vi "Front End.vi"() -> ()   [LabVIEW 2026]
uses:
  <instrlib>/MicroPulse/Public/Data/Datatypes/MP - pulse damping.ctl
  <instrlib>/MicroPulse/Public/Data/Datatypes/MP - frequency filter.ctl
  <instrlib>/MicroPulse/Public/Data/Datatypes/MP - receive parameters.ctl
  <instrlib>/MicroPulse/Public/Data/Datatypes/MP - display gate.ctl
  <instrlib>/MicroPulse/Public/Data/Datatypes/MP - waveform type.ctl
  <instrlib>/MicroPulse/Public/Data/Datatypes/MP - analogue filter.ctl
  <instrlib>/MicroPulse/Public/Data/Datatypes/MP - digital filtering.ctl
  <instrlib>/MicroPulse/Public/Data/Datatypes/MP - high pass filter.ctl
  <instrlib>/MicroPulse/Public/Data/Datatypes/MP - low pass filter.ctl
  <instrlib>/MicroPulse/Public/Data/Datatypes/MP - multi-gate inspection.ctl
  <instrlib>/MicroPulse/Public/Data/Datatypes/MP - multigate inspection gate parameters.ctl
  <instrlib>/MicroPulse/Public/Data/Datatypes/MP - hysteresis level.ctl
  <instrlib>/MicroPulse/Public/Data/Datatypes/MP - multigate mode.ctl
  <instrlib>/MicroPulse/Public/Data/Datatypes/MP - data formatting.ctl
  <instrlib>/MicroPulse/Public/Data/Datatypes/MP - amplitude reporting mode.ctl
  <instrlib>/MicroPulse/Public/Data/Datatypes/MP - averaging.ctl
  <instrlib>/MicroPulse/Public/Data/Datatypes/MP - transmit parameters.ctl
  <instrlib>/MicroPulse/Public/Data/Datatypes/MP - pulser voltage.ctl
  <instrlib>/MicroPulse/Public/Data/Datatypes/TCP config.ctl
  <instrlib>/MicroPulse/Public/Data/Datatypes/MP - sample frequency.ctl
  <instrlib>/MicroPulse/Public/Data/Datatypes/MP - data output format.ctl
  <instrlib>/MicroPulse/Public/Data/Datatypes/MP - test parameters.ctl
  <vilib>/ErrorRing/Error Ring.xnode
  <instrlib>/MicroPulse/MicroPulse_Driver.lvlib
panel:
  in  "Main Tab Control":T1(tab)
  in  "Gain Slider":dbl(slide) caption="Gain (dB)" min=0.0 max=60.0 step=0.25 scale=0.0..60.0
  out "Channel Setup Graph":cluster{"timebase":dbl[], "data":u16[]}[](graph)
  in  "E-Stop Reset":bool
  out "Axis Controls":T2
  in  "Channel Setup Tab Control":enum32{"1", "2", "3", "4", "5", "6", "7"}(tab)
  out "Channel 1 WP/AMP/TOF":T3
  in  "Channel 1 Filter/Rectification/VoS":T5={"Filter"=enum."No change", "Enum"=enum."Rectified Signal", "Velocity of Sound"=6.12}
  in  "Channel 1 A-Scan Window":cluster{"Start":dbl, "Range":dbl}={"Start"=0.0, "Range"=10.0} {"Range" min=0.0 step=5.0; "Start" min=0.0 step=5.0}
  in  "Channel 1 Backwall Gate":T6 {"Threshold" min=0.0 max=100.0 step=1.0; "Length" min=0.0 step=1.0; "Start" min=0.0 step=1.0}
  in  "Channel 1 Flaw Gate":T6 {"Threshold" min=0.0 max=100.0 step=1.0; "Length" min=0.0 step=1.0; "Start" min=0.0 step=1.0}
  in  "Channel 1 Interface":T6 {"Threshold" min=0.0 max=100.0 step=1.0; "Length" min=0.0 step=1.0; "Start" min=0.0 step=1.0}
  in  "Channel 1 PW & DAMP":cluster{"Damping":T7, "Pulse Width":dbl}={"Damping"=enum."149W", "Pulse Width"=80.0} caption="Pulse Width & Damping 1" {"Pulse Width" step=1.0 format="%#_g ns"}
  in  "Channel 2 Filter/Rectification/VoS":T5
  out "Channel 2 WP/AMP/TOF":T3
  in  "Channel 2 A-Scan Window":cluster{"Start":dbl, "Range":dbl}={"Start"=0.0, "Range"=15.0} {"Range" min=0.0 step=1.0; "Start" min=0.0 step=1.0}
  in  "Channel 2 Backwall Gate":T6 {"Threshold" min=0.0 max=100.0 step=1.0; "Length" min=0.0 step=1.0; "Start" min=0.0 step=1.0}
  in  "Channel 2 Flaw Gate":T6 {"Threshold" min=0.0 max=100.0 step=1.0; "Length" min=0.0 step=1.0; "Start" min=0.0 step=1.0}
  in  "Channel 2 Interface":T6 {"Threshold" min=0.0 max=100.0 step=1.0; "Length" min=0.0 step=1.0; "Start" min=0.0 step=1.0}
  in  "Channel 2 PW & DAMP":cluster{"Damping":T7, "Pulse Width":dbl}={"Damping"=enum."149W", "Pulse Width"=80.0} caption="Pulse Width & Damping 1" {"Pulse Width" step=1.0 format="%#_g ns"}
  in  "Channel 3 PW & DAMP":cluster{"Damping":T7, "Pulse Width":dbl}={"Damping"=enum."149W", "Pulse Width"=80.0} caption="Pulse Width & Damping 1" {"Pulse Width" step=1.0 format="%#_g ns"}
  in  "Channel 3 Interface":T6 {"Threshold" min=0.0 max=100.0 step=1.0; "Length" min=0.0 step=1.0; "Start" min=0.0 step=1.0}
  in  "Channel 3 Flaw Gate":T6 {"Threshold" min=0.0 max=100.0 step=1.0; "Length" min=0.0 step=1.0; "Start" min=0.0 step=1.0}
  in  "Channel 3 Backwall Gate":T6 {"Threshold" min=0.0 max=100.0 step=1.0; "Length" min=0.0 step=1.0; "Start" min=0.0 step=1.0}
  in  "Channel 3 A-Scan Window":cluster{"Start":dbl, "Range":dbl}={"Start"=0.0, "Range"=20.0} {"Range" min=0.0 step=1.0; "Start" min=0.0 step=1.0}
  out "Channel 3 WP/AMP/TOF":T3
  in  "Channel 3 Filter/Rectification/VoS":T5
  in  "Channel 4 Filter/Rectification/VoS":T5
  in  "Channel 4 PW & DAMP":cluster{"Damping":T7, "Pulse Width":dbl}={"Damping"=enum."149W", "Pulse Width"=80.0} caption="Pulse Width & Damping 1" {"Pulse Width" step=1.0 format="%#_g ns"}
  in  "Channel 4 Interface":T6 {"Threshold" min=0.0 max=100.0 step=1.0; "Length" min=0.0 step=1.0; "Start" min=0.0 step=1.0}
  in  "Channel 4 Flaw Gate":T6 {"Threshold" min=0.0 max=100.0 step=1.0; "Length" min=0.0 step=1.0; "Start" min=0.0 step=1.0}
  in  "Channel 4 Backwall Gate":T6 {"Threshold" min=0.0 max=100.0 step=1.0; "Length" min=0.0 step=1.0; "Start" min=0.0 step=1.0}
  in  "Channel 4 A-Scan Window":cluster{"Start":dbl, "Range":dbl}={"Start"=0.0, "Range"=25.0} {"Range" min=0.0 step=1.0; "Start" min=0.0 step=1.0}
  out "Channel 4 WP/AMP/TOF":T3
  in  "Channel 5 Filter/Rectification/VoS":T5
  in  "Channel 5 PW & DAMP":cluster{"Damping":T7, "Pulse Width":dbl}={"Damping"=enum."149W", "Pulse Width"=80.0} caption="Pulse Width & Damping 1" {"Pulse Width" step=1.0 format="%#_g ns"}
  in  "Channel 5 Interface":T6 {"Threshold" min=0.0 max=100.0 step=1.0; "Length" min=0.0 step=1.0; "Start" min=0.0 step=1.0}
  in  "Channel 5 Flaw Gate":T6 {"Threshold" min=0.0 max=100.0 step=1.0; "Length" min=0.0 step=1.0; "Start" min=0.0 step=1.0}
  in  "Channel 5 Backwall Gate":T6 {"Threshold" min=0.0 max=100.0 step=1.0; "Length" min=0.0 step=1.0; "Start" min=0.0 step=1.0}
  in  "Channel 5 A-Scan Window":cluster{"Start":dbl, "Range":dbl}={"Start"=0.0, "Range"=30.0} {"Range" min=0.0 step=1.0; "Start" min=0.0 step=1.0}
  out "Channel 5 WP/AMP/TOF":T3
  in  "Channel 6 Filter/Rectification/VoS":T5
  in  "Channel 6 PW & DAMP":cluster{"Damping":T7, "Pulse Width":dbl}={"Damping"=enum."149W", "Pulse Width"=80.0} caption="Pulse Width & Damping 1" {"Pulse Width" step=1.0 format="%#_g ns"}
  in  "Channel 6 Interface":T6 {"Threshold" min=0.0 max=100.0 step=1.0; "Length" min=0.0 step=1.0; "Start" min=0.0 step=1.0}
  in  "Channel 6 Flaw Gate":T6 {"Threshold" min=0.0 max=100.0 step=1.0; "Length" min=0.0 step=1.0; "Start" min=0.0 step=1.0}
  in  "Channel 6 Backwall Gate":T6 {"Threshold" min=0.0 max=100.0 step=1.0; "Length" min=0.0 step=1.0; "Start" min=0.0 step=1.0}
  in  "Channel 6 A-Scan Window":cluster{"Start":dbl, "Range":dbl}={"Start"=0.0, "Range"=35.0} {"Range" min=0.0 step=1.0; "Start" min=0.0 step=1.0}
  out "Channel 6 WP/AMP/TOF":T3
  in  "Channel 7 Filter/Rectification/VoS":T5
  in  "Channel 7 PW & DAMP":cluster{"Damping":T7, "Pulse Width":dbl}={"Damping"=enum."149W", "Pulse Width"=80.0} caption="Pulse Width & Damping 1" {"Pulse Width" step=1.0 format="%#_g ns"}
  in  "Channel 7 Interface":T6 {"Threshold" min=0.0 max=100.0 step=1.0; "Length" min=0.0 step=1.0; "Start" min=0.0 step=1.0}
  in  "Channel 7 Flaw Gate":T6 {"Threshold" min=0.0 max=100.0 step=1.0; "Length" min=0.0 step=1.0; "Start" min=0.0 step=1.0}
  in  "Channel 7 Backwall Gate":T6 {"Threshold" min=0.0 max=100.0 step=1.0; "Length" min=0.0 step=1.0; "Start" min=0.0 step=1.0}
  in  "Channel 7 A-Scan Window":cluster{"Start":dbl, "Range":dbl}={"Start"=0.0, "Range"=40.0} {"Range" min=0.0 step=1.0; "Start" min=0.0 step=1.0}
  out "Channel 7 WP/AMP/TOF":T3
  in  "Channel Select":u16(ring) items=["Channel 1", "Channel 2", "Channel 3", "Channel 4", "Channel 5", "Channel 6", "Channel 7", "Channel 8", "Channel 9"]
  in  "MicroPulse Config Switch":u16(ring) items=["MicroPulse", "Channel 1", "Channel 2", "Channel 3", "Channel 4", "Channel 5", "Channel 6", "Channel 7", "Channel 8", "Channel 9"]
  in  "MicroPulse SysDiag Tab":T8(tab)
  in  "TCP config":T9={"Connection ID"=refnum, "IP address"="10.1.1.2", "host port"=1067, "OC timeout"=-1, "Read timeout"=0, "Write timeout"=0} {"Write timeout" format="%dms"; "Read timeout" format="%dms"; "OC timeout" format="%dms"}
  in  "Sample Frequency":T10
  in  "PRF (Hz)":dbl=50.0
  in  "Mode":T11=enum."8-bit Mode"
  in  "Receive Parameters 1":T12 {"Delay" format="%#_g us"; "Display Gate"."Length" min=0.0 max=64000.0 step=1.0 format="%#_g us"; "Display Gate"."Start" min=0.0 max=64000.0 step=1.0 format="%#_g us"; "Analogue Filtering"."Smoothing" min=1 max=11 step=1; "Gain" min=-6.0 max=70.0 step=0.25 format="%.2fdB"}
  in  "Multi Gate Inspection 1":T19={"Gate 1"={"Start (us)"=0.0, "Length (us)"=0.0, "Threshold"=10, "Enabled?"=TRUE, "Max # Peaks"=0, "Hysteresis"=enum."None", "Mode"=enum."1st Peak in Gate", "Inverted?"=FALSE, "Colour "=6618880}, "Gate 2"={"Start (us)"=0.0, "Length (us)"=0.0, "Threshold"=10, "Enabled?"=TRUE, "Max # Peaks"=0, "Hysteresis"=enum."None", "Mode"=enum."1st Peak in Gate", "Inverted?"=FALSE, "Colour "=16860}, "Gate 3"={"Start (us)"=0.0, "Length (us)"=0.0, "Threshold"=10, "Enabled?"=TRUE, "Max # Peaks"=0, "Hysteresis"=enum."None", "Mode"=enum."1st Peak in Gate", "Inverted?"=FALSE, "Colour "=16711680}, "Gate 4"={"Start (us)"=0.0, "Length (us)"=0.0, "Threshold"=10, "Enabled?"=FALSE, "Max # Peaks"=0, "Hysteresis"=enum."None", "Mode"=enum."1st Peak in Gate", "Inverted?"=FALSE, "Colour "=0}} {"Gate 4"."Max # Peaks" max=64000 step=100; "Gate 4"."Threshold" min=10 max=4095 step=10; "Gate 4"."Length (us)" min=0.0 max=96000.0 step=100.0; "Gate 4"."Start (us)" min=0.0 max=64000.0 step=100.0; "Gate 3"."Max # Peaks" max=64000 step=100; "Gate 3"."Threshold" min=10 max=4095 step=10; "Gate 3"."Length (us)" min=0.0 max=96000.0 step=100.0; "Gate 3"."Start (us)" min=0.0 max=64000.0 step=100.0; "Gate 2"."Max # Peaks" max=64000 step=100; "Gate 2"."Threshold" min=10 max=4095 step=10; "Gate 2"."Length (us)" min=0.0 max=96000.0 step=100.0; "Gate 2"."Start (us)" min=0.0 max=64000.0 step=100.0; "Gate 1"."Max # Peaks" max=64000 step=100; "Gate 1"."Threshold" min=10 max=4095 step=10; "Gate 1"."Length (us)" min=0.0 max=96000.0 step=100.0; "Gate 1"."Start (us)" min=0.0 max=64000.0 step=100.0}
  in  "Data Formatting 1":T23={"Amplitude Mode"=enum."Peaks + Ascan for Multigate", "Averaging"=enum."None", "Coupling Level"=0} {"Coupling Level" max=4095 step=1}
  in  "Transmit Parameters 1":T26 {"Pulse Shape"."Width" min=16 max=1010 step=50 format="%.0fns"}
  in  "Receive Parameters 2":T12 {"Delay" format="%#_g us"; "Display Gate"."Length" min=0.0 max=64000.0 step=1.0 format="%#_g us"; "Display Gate"."Start" min=0.0 max=64000.0 step=1.0 format="%#_g us"; "Analogue Filtering"."Smoothing" min=1 max=11 step=1; "Gain" min=-6.0 max=70.0 step=0.25 format="%.2fdB"}
  in  "Multi Gate Inspection 2":T19={"Gate 1"={"Start (us)"=0.0, "Length (us)"=0.0, "Threshold"=10, "Enabled?"=FALSE, "Max # Peaks"=0, "Hysteresis"=enum."None", "Mode"=enum."1st Peak in Gate", "Inverted?"=FALSE, "Colour "=0}, "Gate 2"={"Start (us)"=0.0, "Length (us)"=0.0, "Threshold"=10, "Enabled?"=FALSE, "Max # Peaks"=0, "Hysteresis"=enum."None", "Mode"=enum."1st Peak in Gate", "Inverted?"=FALSE, "Colour "=0}, "Gate 3"={"Start (us)"=0.0, "Length (us)"=0.0, "Threshold"=10, "Enabled?"=FALSE, "Max # Peaks"=0, "Hysteresis"=enum."None", "Mode"=enum."1st Peak in Gate", "Inverted?"=FALSE, "Colour "=0}, "Gate 4"={"Start (us)"=0.0, "Length (us)"=0.0, "Threshold"=10, "Enabled?"=FALSE, "Max # Peaks"=0, "Hysteresis"=enum."None", "Mode"=enum."1st Peak in Gate", "Inverted?"=FALSE, "Colour "=0}} {"Gate 4"."Max # Peaks" max=64000 step=100; "Gate 4"."Threshold" min=10 max=4095 step=10; "Gate 4"."Length (us)" min=0.0 max=96000.0 step=100.0; "Gate 4"."Start (us)" min=0.0 max=64000.0 step=100.0; "Gate 3"."Max # Peaks" max=64000 step=100; "Gate 3"."Threshold" min=10 max=4095 step=10; "Gate 3"."Length (us)" min=0.0 max=96000.0 step=100.0; "Gate 3"."Start (us)" min=0.0 max=64000.0 step=100.0; "Gate 2"."Max # Peaks" max=64000 step=100; "Gate 2"."Threshold" min=10 max=4095 step=10; "Gate 2"."Length (us)" min=0.0 max=96000.0 step=100.0; "Gate 2"."Start (us)" min=0.0 max=64000.0 step=100.0; "Gate 1"."Max # Peaks" max=64000 step=100; "Gate 1"."Threshold" min=10 max=4095 step=10; "Gate 1"."Length (us)" min=0.0 max=96000.0 step=100.0; "Gate 1"."Start (us)" min=0.0 max=64000.0 step=100.0}
  in  "Data Formatting 2":T23={"Amplitude Mode"=enum."Peaks + Ascan for Multigate", "Averaging"=enum."None", "Coupling Level"=0} {"Coupling Level" max=4095 step=1}
  in  "Transmit Parameters 2":T26 {"Pulse Shape"."Width" min=16 max=1010 step=50 format="%.0fns"}
  in  "Receive Parameters 3":T12 {"Delay" format="%#_g us"; "Display Gate"."Length" min=0.0 max=64000.0 step=1.0 format="%#_g us"; "Display Gate"."Start" min=0.0 max=64000.0 step=1.0 format="%#_g us"; "Analogue Filtering"."Smoothing" min=1 max=11 step=1; "Gain" min=-6.0 max=70.0 step=0.25 format="%.2fdB"}
  in  "Multi Gate Inspection 3":T19={"Gate 1"={"Start (us)"=0.0, "Length (us)"=0.0, "Threshold"=10, "Enabled?"=FALSE, "Max # Peaks"=0, "Hysteresis"=enum."None", "Mode"=enum."1st Peak in Gate", "Inverted?"=FALSE, "Colour "=0}, "Gate 2"={"Start (us)"=0.0, "Length (us)"=0.0, "Threshold"=10, "Enabled?"=FALSE, "Max # Peaks"=0, "Hysteresis"=enum."None", "Mode"=enum."1st Peak in Gate", "Inverted?"=FALSE, "Colour "=0}, "Gate 3"={"Start (us)"=0.0, "Length (us)"=0.0, "Threshold"=10, "Enabled?"=FALSE, "Max # Peaks"=0, "Hysteresis"=enum."None", "Mode"=enum."1st Peak in Gate", "Inverted?"=FALSE, "Colour "=0}, "Gate 4"={"Start (us)"=0.0, "Length (us)"=0.0, "Threshold"=10, "Enabled?"=FALSE, "Max # Peaks"=0, "Hysteresis"=enum."None", "Mode"=enum."1st Peak in Gate", "Inverted?"=FALSE, "Colour "=0}} {"Gate 4"."Max # Peaks" max=64000 step=100; "Gate 4"."Threshold" min=10 max=4095 step=10; "Gate 4"."Length (us)" min=0.0 max=96000.0 step=100.0; "Gate 4"."Start (us)" min=0.0 max=64000.0 step=100.0; "Gate 3"."Max # Peaks" max=64000 step=100; "Gate 3"."Threshold" min=10 max=4095 step=10; "Gate 3"."Length (us)" min=0.0 max=96000.0 step=100.0; "Gate 3"."Start (us)" min=0.0 max=64000.0 step=100.0; "Gate 2"."Max # Peaks" max=64000 step=100; "Gate 2"."Threshold" min=10 max=4095 step=10; "Gate 2"."Length (us)" min=0.0 max=96000.0 step=100.0; "Gate 2"."Start (us)" min=0.0 max=64000.0 step=100.0; "Gate 1"."Max # Peaks" max=64000 step=100; "Gate 1"."Threshold" min=10 max=4095 step=10; "Gate 1"."Length (us)" min=0.0 max=96000.0 step=100.0; "Gate 1"."Start (us)" min=0.0 max=64000.0 step=100.0}
  in  "Data Formatting 3":T23={"Amplitude Mode"=enum."Peaks + Ascan for Multigate", "Averaging"=enum."None", "Coupling Level"=0} {"Coupling Level" max=4095 step=1}
  in  "Transmit Parameters 3":T26 {"Pulse Shape"."Width" min=16 max=1010 step=50 format="%.0fns"}
  in  "Receive Parameters 4":T12 {"Delay" format="%#_g us"; "Display Gate"."Length" min=0.0 max=64000.0 step=1.0 format="%#_g us"; "Display Gate"."Start" min=0.0 max=64000.0 step=1.0 format="%#_g us"; "Analogue Filtering"."Smoothing" min=1 max=11 step=1; "Gain" min=-6.0 max=70.0 step=0.25 format="%.2fdB"}
  in  "Multi Gate Inspection 4":T19={"Gate 1"={"Start (us)"=0.0, "Length (us)"=0.0, "Threshold"=10, "Enabled?"=FALSE, "Max # Peaks"=0, "Hysteresis"=enum."None", "Mode"=enum."1st Peak in Gate", "Inverted?"=FALSE, "Colour "=0}, "Gate 2"={"Start (us)"=0.0, "Length (us)"=0.0, "Threshold"=10, "Enabled?"=FALSE, "Max # Peaks"=0, "Hysteresis"=enum."None", "Mode"=enum."1st Peak in Gate", "Inverted?"=FALSE, "Colour "=0}, "Gate 3"={"Start (us)"=0.0, "Length (us)"=0.0, "Threshold"=10, "Enabled?"=FALSE, "Max # Peaks"=0, "Hysteresis"=enum."None", "Mode"=enum."1st Peak in Gate", "Inverted?"=FALSE, "Colour "=0}, "Gate 4"={"Start (us)"=0.0, "Length (us)"=0.0, "Threshold"=10, "Enabled?"=FALSE, "Max # Peaks"=0, "Hysteresis"=enum."None", "Mode"=enum."1st Peak in Gate", "Inverted?"=FALSE, "Colour "=0}} {"Gate 4"."Max # Peaks" max=64000 step=100; "Gate 4"."Threshold" min=10 max=4095 step=10; "Gate 4"."Length (us)" min=0.0 max=96000.0 step=100.0; "Gate 4"."Start (us)" min=0.0 max=64000.0 step=100.0; "Gate 3"."Max # Peaks" max=64000 step=100; "Gate 3"."Threshold" min=10 max=4095 step=10; "Gate 3"."Length (us)" min=0.0 max=96000.0 step=100.0; "Gate 3"."Start (us)" min=0.0 max=64000.0 step=100.0; "Gate 2"."Max # Peaks" max=64000 step=100; "Gate 2"."Threshold" min=10 max=4095 step=10; "Gate 2"."Length (us)" min=0.0 max=96000.0 step=100.0; "Gate 2"."Start (us)" min=0.0 max=64000.0 step=100.0; "Gate 1"."Max # Peaks" max=64000 step=100; "Gate 1"."Threshold" min=10 max=4095 step=10; "Gate 1"."Length (us)" min=0.0 max=96000.0 step=100.0; "Gate 1"."Start (us)" min=0.0 max=64000.0 step=100.0}
  in  "Data Formatting 4":T23={"Amplitude Mode"=enum."Peaks + Ascan for Multigate", "Averaging"=enum."None", "Coupling Level"=0} {"Coupling Level" max=4095 step=1}
  in  "Transmit Parameters 4":T26 {"Pulse Shape"."Width" min=16 max=1010 step=50 format="%.0fns"}
  in  "Receive Parameters 5":T12 {"Delay" format="%#_g us"; "Display Gate"."Length" min=0.0 max=64000.0 step=1.0 format="%#_g us"; "Display Gate"."Start" min=0.0 max=64000.0 step=1.0 format="%#_g us"; "Analogue Filtering"."Smoothing" min=1 max=11 step=1; "Gain" min=-6.0 max=70.0 step=0.25 format="%.2fdB"}
  in  "Multi Gate Inspection 5":T19={"Gate 1"={"Start (us)"=0.0, "Length (us)"=0.0, "Threshold"=10, "Enabled?"=FALSE, "Max # Peaks"=0, "Hysteresis"=enum."None", "Mode"=enum."1st Peak in Gate", "Inverted?"=FALSE, "Colour "=0}, "Gate 2"={"Start (us)"=0.0, "Length (us)"=0.0, "Threshold"=10, "Enabled?"=FALSE, "Max # Peaks"=0, "Hysteresis"=enum."None", "Mode"=enum."1st Peak in Gate", "Inverted?"=FALSE, "Colour "=0}, "Gate 3"={"Start (us)"=0.0, "Length (us)"=0.0, "Threshold"=10, "Enabled?"=FALSE, "Max # Peaks"=0, "Hysteresis"=enum."None", "Mode"=enum."1st Peak in Gate", "Inverted?"=FALSE, "Colour "=0}, "Gate 4"={"Start (us)"=0.0, "Length (us)"=0.0, "Threshold"=10, "Enabled?"=FALSE, "Max # Peaks"=0, "Hysteresis"=enum."None", "Mode"=enum."1st Peak in Gate", "Inverted?"=FALSE, "Colour "=0}} {"Gate 4"."Max # Peaks" max=64000 step=100; "Gate 4"."Threshold" min=10 max=4095 step=10; "Gate 4"."Length (us)" min=0.0 max=96000.0 step=100.0; "Gate 4"."Start (us)" min=0.0 max=64000.0 step=100.0; "Gate 3"."Max # Peaks" max=64000 step=100; "Gate 3"."Threshold" min=10 max=4095 step=10; "Gate 3"."Length (us)" min=0.0 max=96000.0 step=100.0; "Gate 3"."Start (us)" min=0.0 max=64000.0 step=100.0; "Gate 2"."Max # Peaks" max=64000 step=100; "Gate 2"."Threshold" min=10 max=4095 step=10; "Gate 2"."Length (us)" min=0.0 max=96000.0 step=100.0; "Gate 2"."Start (us)" min=0.0 max=64000.0 step=100.0; "Gate 1"."Max # Peaks" max=64000 step=100; "Gate 1"."Threshold" min=10 max=4095 step=10; "Gate 1"."Length (us)" min=0.0 max=96000.0 step=100.0; "Gate 1"."Start (us)" min=0.0 max=64000.0 step=100.0}
  in  "Data Formatting 5":T23={"Amplitude Mode"=enum."Peaks + Ascan for Multigate", "Averaging"=enum."None", "Coupling Level"=0} {"Coupling Level" max=4095 step=1}
  in  "Transmit Parameters 5":T26 {"Pulse Shape"."Width" min=16 max=1010 step=50 format="%.0fns"}
  in  "Receive Parameters 6":T12 {"Delay" format="%#_g us"; "Display Gate"."Length" min=0.0 max=64000.0 step=1.0 format="%#_g us"; "Display Gate"."Start" min=0.0 max=64000.0 step=1.0 format="%#_g us"; "Analogue Filtering"."Smoothing" min=1 max=11 step=1; "Gain" min=-6.0 max=70.0 step=0.25 format="%.2fdB"}
  in  "Multi Gate Inspection 6":T19={"Gate 1"={"Start (us)"=0.0, "Length (us)"=0.0, "Threshold"=10, "Enabled?"=FALSE, "Max # Peaks"=0, "Hysteresis"=enum."None", "Mode"=enum."1st Peak in Gate", "Inverted?"=FALSE, "Colour "=0}, "Gate 2"={"Start (us)"=0.0, "Length (us)"=0.0, "Threshold"=10, "Enabled?"=FALSE, "Max # Peaks"=0, "Hysteresis"=enum."None", "Mode"=enum."1st Peak in Gate", "Inverted?"=FALSE, "Colour "=0}, "Gate 3"={"Start (us)"=0.0, "Length (us)"=0.0, "Threshold"=10, "Enabled?"=FALSE, "Max # Peaks"=0, "Hysteresis"=enum."None", "Mode"=enum."1st Peak in Gate", "Inverted?"=FALSE, "Colour "=0}, "Gate 4"={"Start (us)"=0.0, "Length (us)"=0.0, "Threshold"=10, "Enabled?"=FALSE, "Max # Peaks"=0, "Hysteresis"=enum."None", "Mode"=enum."1st Peak in Gate", "Inverted?"=FALSE, "Colour "=0}} {"Gate 4"."Max # Peaks" max=64000 step=100; "Gate 4"."Threshold" min=10 max=4095 step=10; "Gate 4"."Length (us)" min=0.0 max=96000.0 step=100.0; "Gate 4"."Start (us)" min=0.0 max=64000.0 step=100.0; "Gate 3"."Max # Peaks" max=64000 step=100; "Gate 3"."Threshold" min=10 max=4095 step=10; "Gate 3"."Length (us)" min=0.0 max=96000.0 step=100.0; "Gate 3"."Start (us)" min=0.0 max=64000.0 step=100.0; "Gate 2"."Max # Peaks" max=64000 step=100; "Gate 2"."Threshold" min=10 max=4095 step=10; "Gate 2"."Length (us)" min=0.0 max=96000.0 step=100.0; "Gate 2"."Start (us)" min=0.0 max=64000.0 step=100.0; "Gate 1"."Max # Peaks" max=64000 step=100; "Gate 1"."Threshold" min=10 max=4095 step=10; "Gate 1"."Length (us)" min=0.0 max=96000.0 step=100.0; "Gate 1"."Start (us)" min=0.0 max=64000.0 step=100.0}
  in  "Data Formatting 6":T23={"Amplitude Mode"=enum."Peaks + Ascan for Multigate", "Averaging"=enum."None", "Coupling Level"=0} {"Coupling Level" max=4095 step=1}
  in  "Transmit Parameters 6":T26 {"Pulse Shape"."Width" min=16 max=1010 step=50 format="%.0fns"}
  in  "Receive Parameters 7":T12 {"Delay" format="%#_g us"; "Display Gate"."Length" min=0.0 max=64000.0 step=1.0 format="%#_g us"; "Display Gate"."Start" min=0.0 max=64000.0 step=1.0 format="%#_g us"; "Analogue Filtering"."Smoothing" min=1 max=11 step=1; "Gain" min=-6.0 max=70.0 step=0.25 format="%.2fdB"}
  in  "Multi Gate Inspection 7":T19={"Gate 1"={"Start (us)"=0.0, "Length (us)"=0.0, "Threshold"=10, "Enabled?"=FALSE, "Max # Peaks"=0, "Hysteresis"=enum."None", "Mode"=enum."1st Peak in Gate", "Inverted?"=FALSE, "Colour "=0}, "Gate 2"={"Start (us)"=0.0, "Length (us)"=0.0, "Threshold"=10, "Enabled?"=FALSE, "Max # Peaks"=0, "Hysteresis"=enum."None", "Mode"=enum."1st Peak in Gate", "Inverted?"=FALSE, "Colour "=0}, "Gate 3"={"Start (us)"=0.0, "Length (us)"=0.0, "Threshold"=10, "Enabled?"=FALSE, "Max # Peaks"=0, "Hysteresis"=enum."None", "Mode"=enum."1st Peak in Gate", "Inverted?"=FALSE, "Colour "=0}, "Gate 4"={"Start (us)"=0.0, "Length (us)"=0.0, "Threshold"=10, "Enabled?"=FALSE, "Max # Peaks"=0, "Hysteresis"=enum."None", "Mode"=enum."1st Peak in Gate", "Inverted?"=FALSE, "Colour "=0}} {"Gate 4"."Max # Peaks" max=64000 step=100; "Gate 4"."Threshold" min=10 max=4095 step=10; "Gate 4"."Length (us)" min=0.0 max=96000.0 step=100.0; "Gate 4"."Start (us)" min=0.0 max=64000.0 step=100.0; "Gate 3"."Max # Peaks" max=64000 step=100; "Gate 3"."Threshold" min=10 max=4095 step=10; "Gate 3"."Length (us)" min=0.0 max=96000.0 step=100.0; "Gate 3"."Start (us)" min=0.0 max=64000.0 step=100.0; "Gate 2"."Max # Peaks" max=64000 step=100; "Gate 2"."Threshold" min=10 max=4095 step=10; "Gate 2"."Length (us)" min=0.0 max=96000.0 step=100.0; "Gate 2"."Start (us)" min=0.0 max=64000.0 step=100.0; "Gate 1"."Max # Peaks" max=64000 step=100; "Gate 1"."Threshold" min=10 max=4095 step=10; "Gate 1"."Length (us)" min=0.0 max=96000.0 step=100.0; "Gate 1"."Start (us)" min=0.0 max=64000.0 step=100.0}
  in  "Data Formatting 7":T23={"Amplitude Mode"=enum."Peaks + Ascan for Multigate", "Averaging"=enum."None", "Coupling Level"=0} {"Coupling Level" max=4095 step=1}
  in  "Transmit Parameters 7":T26 {"Pulse Shape"."Width" min=16 max=1010 step=50 format="%.0fns"}
  in  "Receive Parameters 8":T12 {"Delay" format="%#_g us"; "Display Gate"."Length" min=0.0 max=64000.0 step=1.0 format="%#_g us"; "Display Gate"."Start" min=0.0 max=64000.0 step=1.0 format="%#_g us"; "Analogue Filtering"."Smoothing" min=1 max=11 step=1; "Gain" min=-6.0 max=70.0 step=0.25 format="%.2fdB"}
  in  "Multi Gate Inspection 8":T19={"Gate 1"={"Start (us)"=0.0, "Length (us)"=0.0, "Threshold"=10, "Enabled?"=FALSE, "Max # Peaks"=0, "Hysteresis"=enum."None", "Mode"=enum."1st Peak in Gate", "Inverted?"=FALSE, "Colour "=0}, "Gate 2"={"Start (us)"=0.0, "Length (us)"=0.0, "Threshold"=10, "Enabled?"=FALSE, "Max # Peaks"=0, "Hysteresis"=enum."None", "Mode"=enum."1st Peak in Gate", "Inverted?"=FALSE, "Colour "=0}, "Gate 3"={"Start (us)"=0.0, "Length (us)"=0.0, "Threshold"=10, "Enabled?"=FALSE, "Max # Peaks"=0, "Hysteresis"=enum."None", "Mode"=enum."1st Peak in Gate", "Inverted?"=FALSE, "Colour "=0}, "Gate 4"={"Start (us)"=0.0, "Length (us)"=0.0, "Threshold"=10, "Enabled?"=FALSE, "Max # Peaks"=0, "Hysteresis"=enum."None", "Mode"=enum."1st Peak in Gate", "Inverted?"=FALSE, "Colour "=0}} {"Gate 4"."Max # Peaks" max=64000 step=100; "Gate 4"."Threshold" min=10 max=4095 step=10; "Gate 4"."Length (us)" min=0.0 max=96000.0 step=100.0; "Gate 4"."Start (us)" min=0.0 max=64000.0 step=100.0; "Gate 3"."Max # Peaks" max=64000 step=100; "Gate 3"."Threshold" min=10 max=4095 step=10; "Gate 3"."Length (us)" min=0.0 max=96000.0 step=100.0; "Gate 3"."Start (us)" min=0.0 max=64000.0 step=100.0; "Gate 2"."Max # Peaks" max=64000 step=100; "Gate 2"."Threshold" min=10 max=4095 step=10; "Gate 2"."Length (us)" min=0.0 max=96000.0 step=100.0; "Gate 2"."Start (us)" min=0.0 max=64000.0 step=100.0; "Gate 1"."Max # Peaks" max=64000 step=100; "Gate 1"."Threshold" min=10 max=4095 step=10; "Gate 1"."Length (us)" min=0.0 max=96000.0 step=100.0; "Gate 1"."Start (us)" min=0.0 max=64000.0 step=100.0}
  in  "Data Formatting 8":T23={"Amplitude Mode"=enum."Peaks + Ascan for Multigate", "Averaging"=enum."None", "Coupling Level"=0} {"Coupling Level" max=4095 step=1}
  in  "Transmit Parameters 8":T26 {"Pulse Shape"."Width" min=16 max=1010 step=50 format="%.0fns"}
  in  "Receive Parameters 9":T12 {"Delay" format="%#_g us"; "Display Gate"."Length" min=0.0 max=64000.0 step=1.0 format="%#_g us"; "Display Gate"."Start" min=0.0 max=64000.0 step=1.0 format="%#_g us"; "Analogue Filtering"."Smoothing" min=1 max=11 step=1; "Gain" min=-6.0 max=70.0 step=0.25 format="%.2fdB"}
  in  "Multi Gate Inspection 9":T19={"Gate 1"={"Start (us)"=0.0, "Length (us)"=0.0, "Threshold"=10, "Enabled?"=FALSE, "Max # Peaks"=0, "Hysteresis"=enum."None", "Mode"=enum."1st Peak in Gate", "Inverted?"=FALSE, "Colour "=0}, "Gate 2"={"Start (us)"=0.0, "Length (us)"=0.0, "Threshold"=10, "Enabled?"=FALSE, "Max # Peaks"=0, "Hysteresis"=enum."None", "Mode"=enum."1st Peak in Gate", "Inverted?"=FALSE, "Colour "=0}, "Gate 3"={"Start (us)"=0.0, "Length (us)"=0.0, "Threshold"=10, "Enabled?"=FALSE, "Max # Peaks"=0, "Hysteresis"=enum."None", "Mode"=enum."1st Peak in Gate", "Inverted?"=FALSE, "Colour "=0}, "Gate 4"={"Start (us)"=0.0, "Length (us)"=0.0, "Threshold"=10, "Enabled?"=FALSE, "Max # Peaks"=0, "Hysteresis"=enum."None", "Mode"=enum."1st Peak in Gate", "Inverted?"=FALSE, "Colour "=0}} {"Gate 4"."Max # Peaks" max=64000 step=100; "Gate 4"."Threshold" min=10 max=4095 step=10; "Gate 4"."Length (us)" min=0.0 max=96000.0 step=100.0; "Gate 4"."Start (us)" min=0.0 max=64000.0 step=100.0; "Gate 3"."Max # Peaks" max=64000 step=100; "Gate 3"."Threshold" min=10 max=4095 step=10; "Gate 3"."Length (us)" min=0.0 max=96000.0 step=100.0; "Gate 3"."Start (us)" min=0.0 max=64000.0 step=100.0; "Gate 2"."Max # Peaks" max=64000 step=100; "Gate 2"."Threshold" min=10 max=4095 step=10; "Gate 2"."Length (us)" min=0.0 max=96000.0 step=100.0; "Gate 2"."Start (us)" min=0.0 max=64000.0 step=100.0; "Gate 1"."Max # Peaks" max=64000 step=100; "Gate 1"."Threshold" min=10 max=4095 step=10; "Gate 1"."Length (us)" min=0.0 max=96000.0 step=100.0; "Gate 1"."Start (us)" min=0.0 max=64000.0 step=100.0}
  in  "Data Formatting 9":T23={"Amplitude Mode"=enum."Peaks + Ascan for Multigate", "Averaging"=enum."None", "Coupling Level"=0} {"Coupling Level" max=4095 step=1}
  in  "Transmit Parameters 9":T26 {"Pulse Shape"."Width" min=16 max=1010 step=50 format="%.0fns"}
  in  "stop":bool
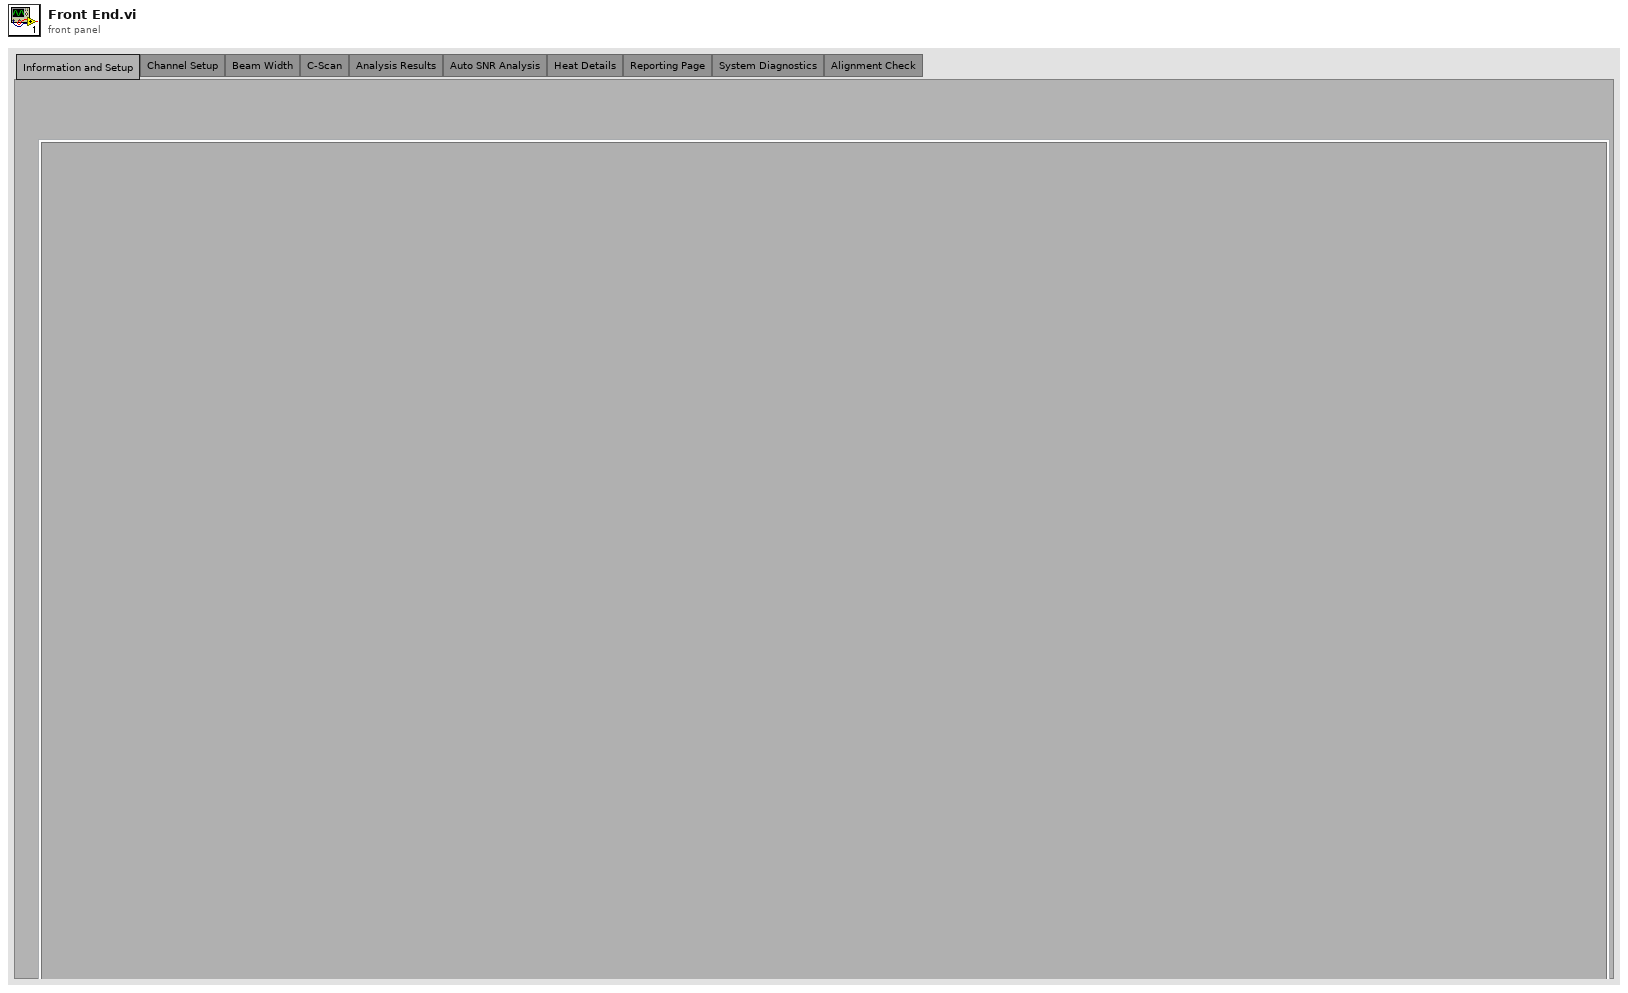
[diagram p1: front panel]
types:
  T1 = enum32{"Information and Setup", "Channel Setup", "Beam Width", "C-Scan", "Analysis Results", "Auto SNR Analysis", "Heat Details", "Reporting Page", "System Diagnostics", "Alignment Check"}
  T2 = cluster{"Buttons":cluster{"Datum":bool, "Move to Bar":bool, "Move to Home":bool}, "X Axis":cluster{"Calculated X Value":dbl, "Encoder X Value":dbl, "X Axis Movement Buttons":cluster{"Left":bool, "Right":bool, "Go To":bool, "Stop":bool}}, "Y Axis":cluster{"Encoder Y Value":dbl, "Y Axis Movement Buttons":cluster{"Left":bool, "Right":bool, "Go To":bool, "Stop":bool}, "Z Axis":cluster{"Encoder Z Value":dbl, "Z Axis Movement Buttons":cluster{"Left":bool, "Right":bool, "Go To":bool, "Stop":bool}}, "Rotate Axis":cluster{"Calculated Rotate Value":dbl, "Encoder Rotate Value":dbl, "Rotate Axis Movement Buttons":cluster{"Left":bool, "Right":bool, "Go To":bool, "Stop":bool}}, "Pitch Axis":cluster{"Encoder Pitch Value":dbl, "Pitch Axis Movement Buttons":cluster{"Left":bool, "Right":bool, "Go To":bool, "Stop":bool}}, "Roll Axis":cluster{"Encoder Roll Value":dbl, "Roll Axis Movement Buttons":cluster{"Left":bool, "Right":bool, "Go To":bool, "Stop":bool}}}}
  T3 = cluster{"Water Path":dbl, "Gate Amplitude":dbl, "Gate TOF":dbl}
  T4 = typedef "MicroPulse_Driver.lvlib/MP - frequency filter.ctl" = enum16{"No change", "1MHz Bandpass", "2MHz Bandpass", "4MHz Bandpass", "5MHz Bandpass", "10MHz Bandpass", "2.5-18MHz Broadband", "0.75-12MHz  Broadband", "0.5MHz Bandpass", "5MHz 2nd Order TOFD", "10MHz 2nd Order TOFD", "3.0-25MHz Broadband", "3.0-30MHz Broadband"}
  T5 = cluster{"Filter":T4, "Enum":enum16{"Rectified Signal", "RF Signal", "+Half Wave", "-Half Wave"}, "Velocity of Sound":dbl}
  T6 = cluster{"Start":dbl, "Length":dbl, "Threshold":dbl}
  T7 = typedef "MicroPulse_Driver.lvlib/MP - pulse damping.ctl" = enum16{"660W", "458W", "220W", "149W", "102W", "82W", "63W", "51W"}
  T8 = enum32{"MicroPulse", "Channel 1", "Channel 2", "Channel 3", "Channel 4", "Channel 5", "Channel 6", "Channel 7", "Channel 8", "Channel 9"}
  T9 = typedef "MicroPulse_Driver.lvlib/TCP config.ctl" = cluster{"Connection ID":refnum<k5>, "IP address":string, "host port":u16, "OC timeout":i32, "Read timeout":i32, "Write timeout":i32}
  T10 = typedef "MicroPulse_Driver.lvlib/MP - sample frequency.ctl" = enum16{"Use Default", "200MHz (LT2 only)", "100MHz", "50MHz", "25MHz", "10MHz"}
  T11 = typedef "MicroPulse_Driver.lvlib/MP - data output format.ctl" = enum16{"", "8-bit Mode", "10-bit Mode", "12-bit Mode", "16-bit Mode", "8-bit Log Mode", "12-bit Packed Mode"}
  T12 = typedef "MicroPulse_Driver.lvlib/MP - receive parameters.ctl" = cluster{"Display Gate":T13, "Delay":dbl, "Waveform Type":T14, "Gain":dbl, "Analogue Filtering":T15, "Digital Filtering":T16}
  T13 = typedef "MicroPulse_Driver.lvlib/MP - display gate.ctl" = cluster{"Start":dbl, "Length":dbl}
  T14 = typedef "MicroPulse_Driver.lvlib/MP - waveform type.ctl" = enum16{"Rectified Signal", "RF Signal", "+Half Wave", "-Half Wave"}
  T15 = typedef "MicroPulse_Driver.lvlib/MP - analogue filter.ctl" = cluster{"Bandpass":T4, "Smoothing":u16}
  T16 = typedef "MicroPulse_Driver.lvlib/MP - digital filtering.ctl" = cluster{"High Pass Filter":T17, "Low Pass Filter":T18}
  T17 = typedef "MicroPulse_Driver.lvlib/MP - high pass filter.ctl" = enum16{"None", "0.7MHz", "1.5MHz", "4.0MHz", "7.5MHz", "10.0MHz", "User Defined"}
  T18 = typedef "MicroPulse_Driver.lvlib/MP - low pass filter.ctl" = enum16{"None", "1.8MHz", "3.0MHz", "6.0MHz", "8.0MHz", "12.0MHz", "User Defined"}
  T19 = typedef "MicroPulse_Driver.lvlib/MP - multi-gate inspection.ctl" = cluster{"Gate 1":T20, "Gate 2":T20, "Gate 3":T20, "Gate 4":T20}
  T20 = typedef "MicroPulse_Driver.lvlib/MP - multigate inspection gate parameters.ctl" = cluster{"Start (us)":dbl, "Length (us)":dbl, "Threshold":u16, "Enabled?":bool, "Max # Peaks":u16, "Hysteresis":T21, "Mode":T22, "Inverted?":bool, "Colour ":u32}
  T21 = typedef "MicroPulse_Driver.lvlib/MP - hysteresis level.ctl" = enum16{"None", "3dB", "6dB", "9dB", "12dB"}
  T22 = typedef "MicroPulse_Driver.lvlib/MP - multigate mode.ctl" = enum16{"1st Peak in Gate", "Largest Peak In Gate", "All Peaks In Gate", "1st Threshold Crossing"}
  T23 = typedef "MicroPulse_Driver.lvlib/MP - data formatting.ctl" = cluster{"Amplitude Mode":T24, "Averaging":T25, "Coupling Level":u32}
  T24 = typedef "MicroPulse_Driver.lvlib/MP - amplitude reporting mode.ctl" = enum16{"1st Peak in gate", "Maximum Peak in gate", "All Peaks", "Ascan Data", "1st Threshold Crossing Peak", "Ascan + Peaks", "All Peaks for Multigate", "Peaks + Ascan for Multigate", "Peaks + P_Ascan for Multigate", "Full Matrix Capture"}
  T25 = typedef "MicroPulse_Driver.lvlib/MP - averaging.ctl" = enum16{"None", "2", "4", "8", "16", "32", "64", "128", "256"}
  T26 = typedef "MicroPulse_Driver.lvlib/MP - transmit parameters.ctl" = cluster{"Pulse Voltage":T27, "Pulse Shape":cluster{"Damping":T7, "Width":u32}}
  T27 = typedef "MicroPulse_Driver.lvlib/MP - pulser voltage.ctl" = enum16{"50V", "100V", "150V", "200V", "250V", "300V"}
  T28 = enum16{"Channel 1", "Channel 2", "Channel 3", "Channel 4", "Channel 5", "Channel 6", "Channel 7", "Channel 8", "Channel 9"}
  T29 = enum16{"Init", "Init HW", "Main", "Error", "Shutdown"}
  T30 = typedef "MicroPulse_Driver.lvlib/MP - test parameters.ctl" = cluster{"Test No.":u32, "Tx Channel":u32, "Rx Channel":u32}
  T31 = enum16{"Rectified Signal", "RF Signal", "+Half Wave", "-Half Wave"}
  T32 = typedef "MicroPulse_Driver.lvlib/MP - scan data info.ctl" = cluster{"Message Header":u16, "Error Message":u16, "Test No.":u32, "Channel No.":u8, "Sweep No.":u32, "Gate No.":u32, "DOF":T11, "retain data":T33, "scan data":u16[], "scan length":i32, "scan index":i32, "peak data":cluster{"timebase":u16[], "data":u16[]}, "#peaks":i32, "PRF":dbl, "IP":cluster{"Axis No.":u8, "Location":u32, "MIP location":u32, "MIP?":bool}, "echo range":u16, "ETG":bool, "CAL 0 complete":bool, "Axis Positions":T34}
  T33 = typedef "MicroPulse_Driver.lvlib/MP - retain scan.ctl" = enum16{"None", "Ascan", "Peaks"}
  T34 = typedef "MicroPulse_Driver.lvlib/MP - axis positions (LLC).ctl" = cluster{"Axis 1":u32, "Axis 2":u32, "Axis 3":u32, "Axis 4":u32, "Status":u8}
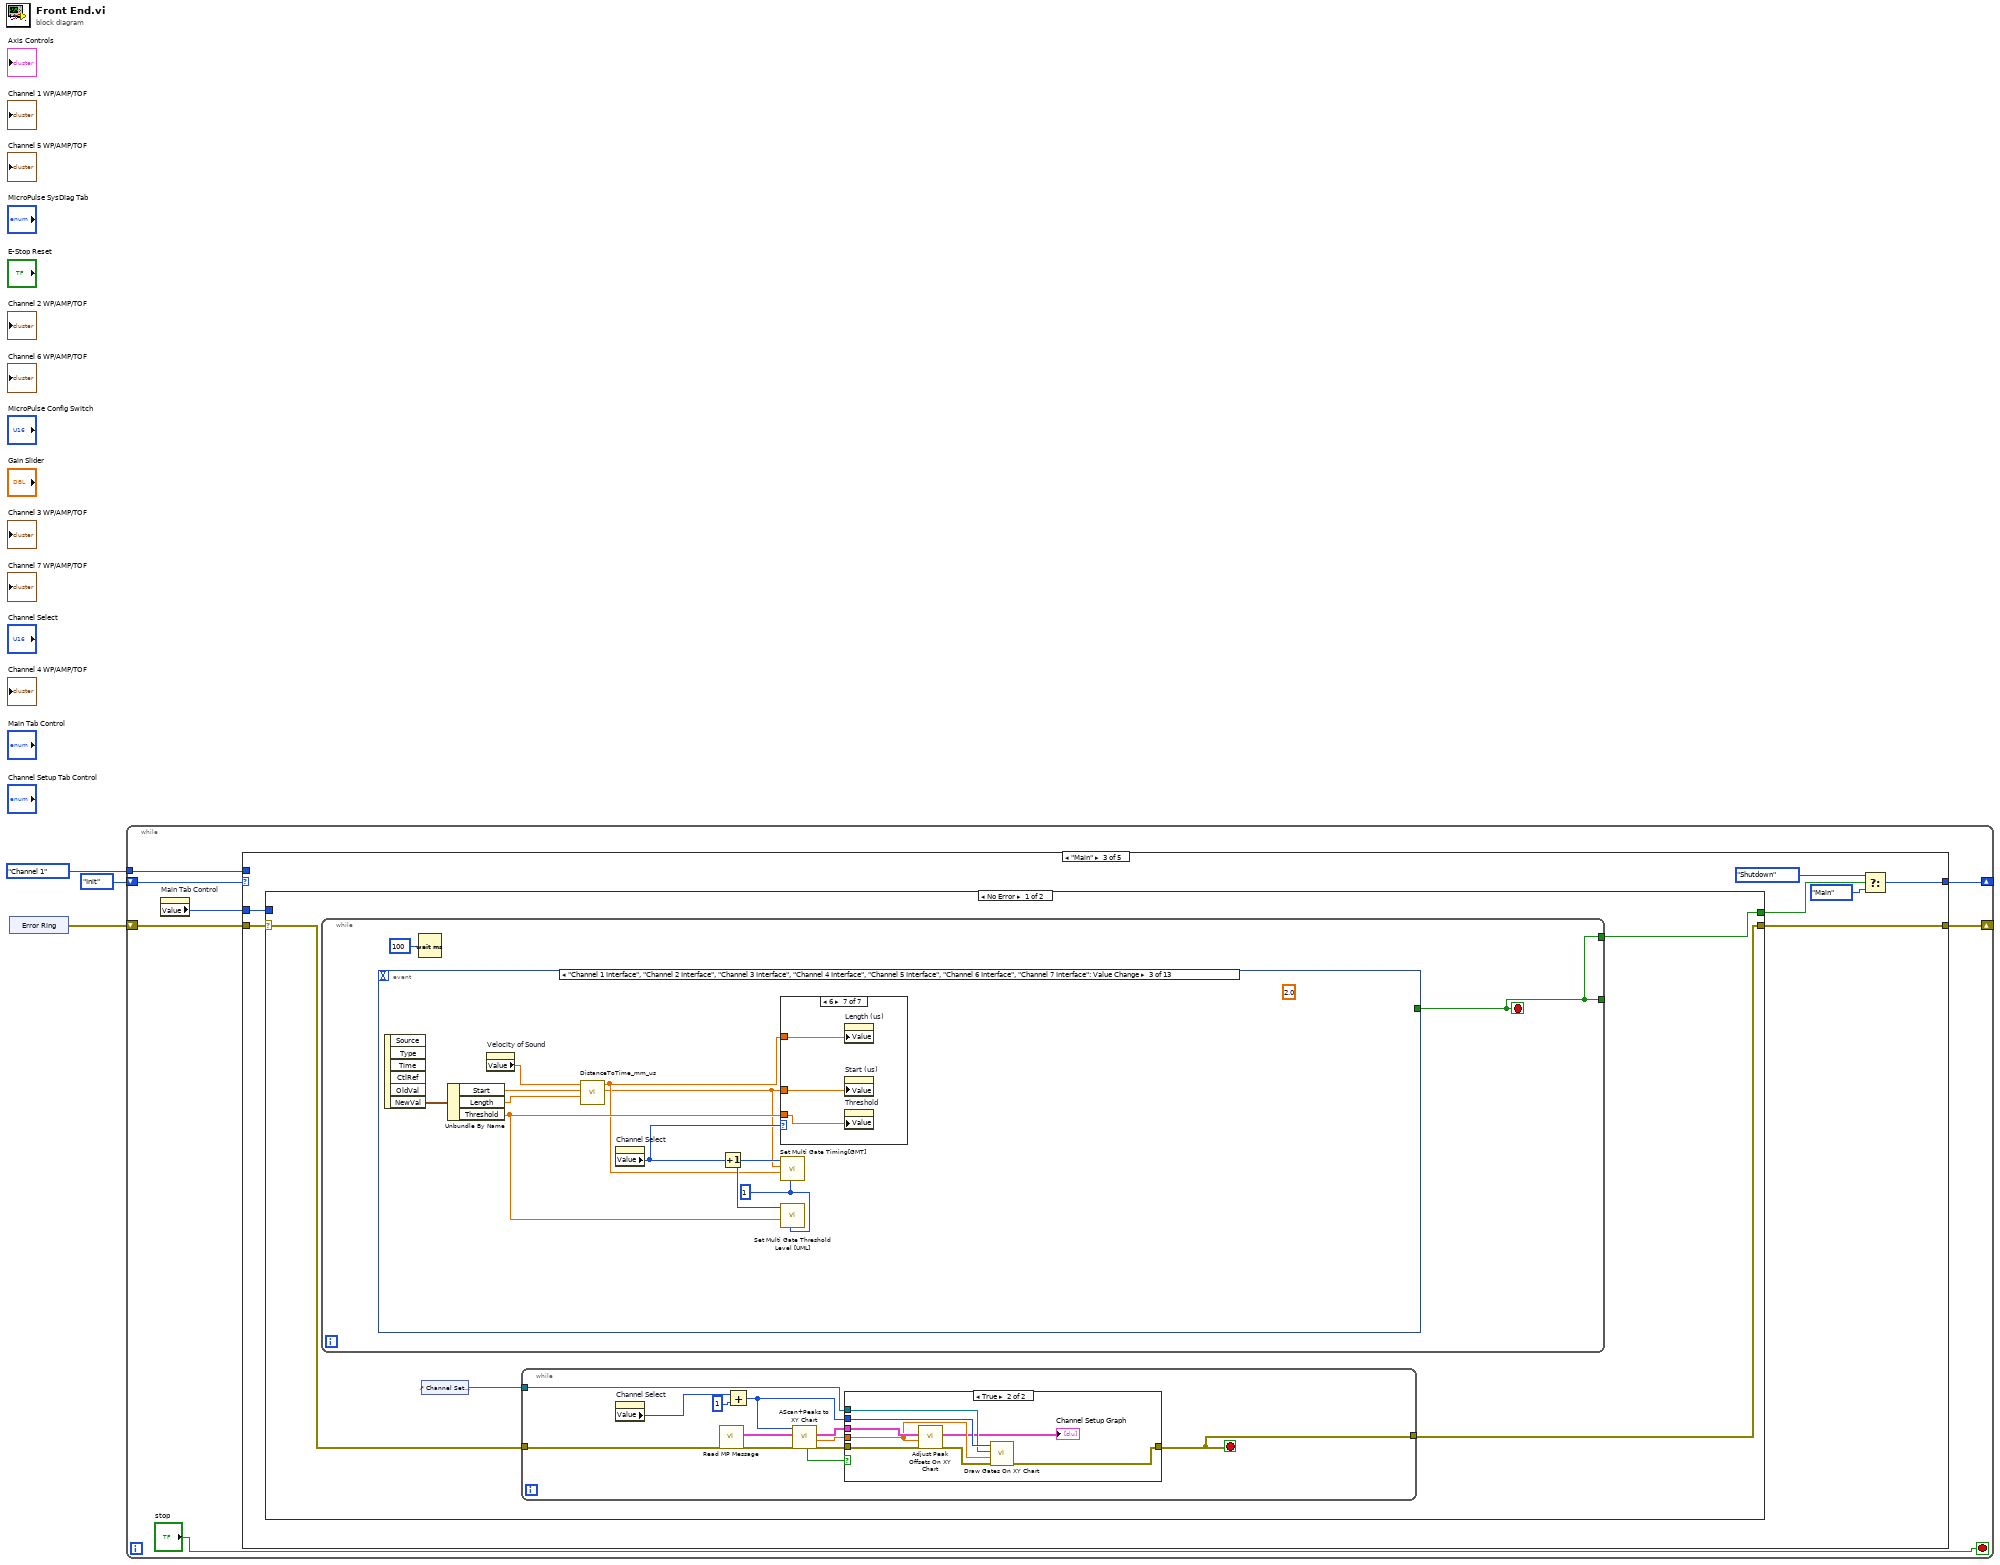
[diagram p0: block diagram]
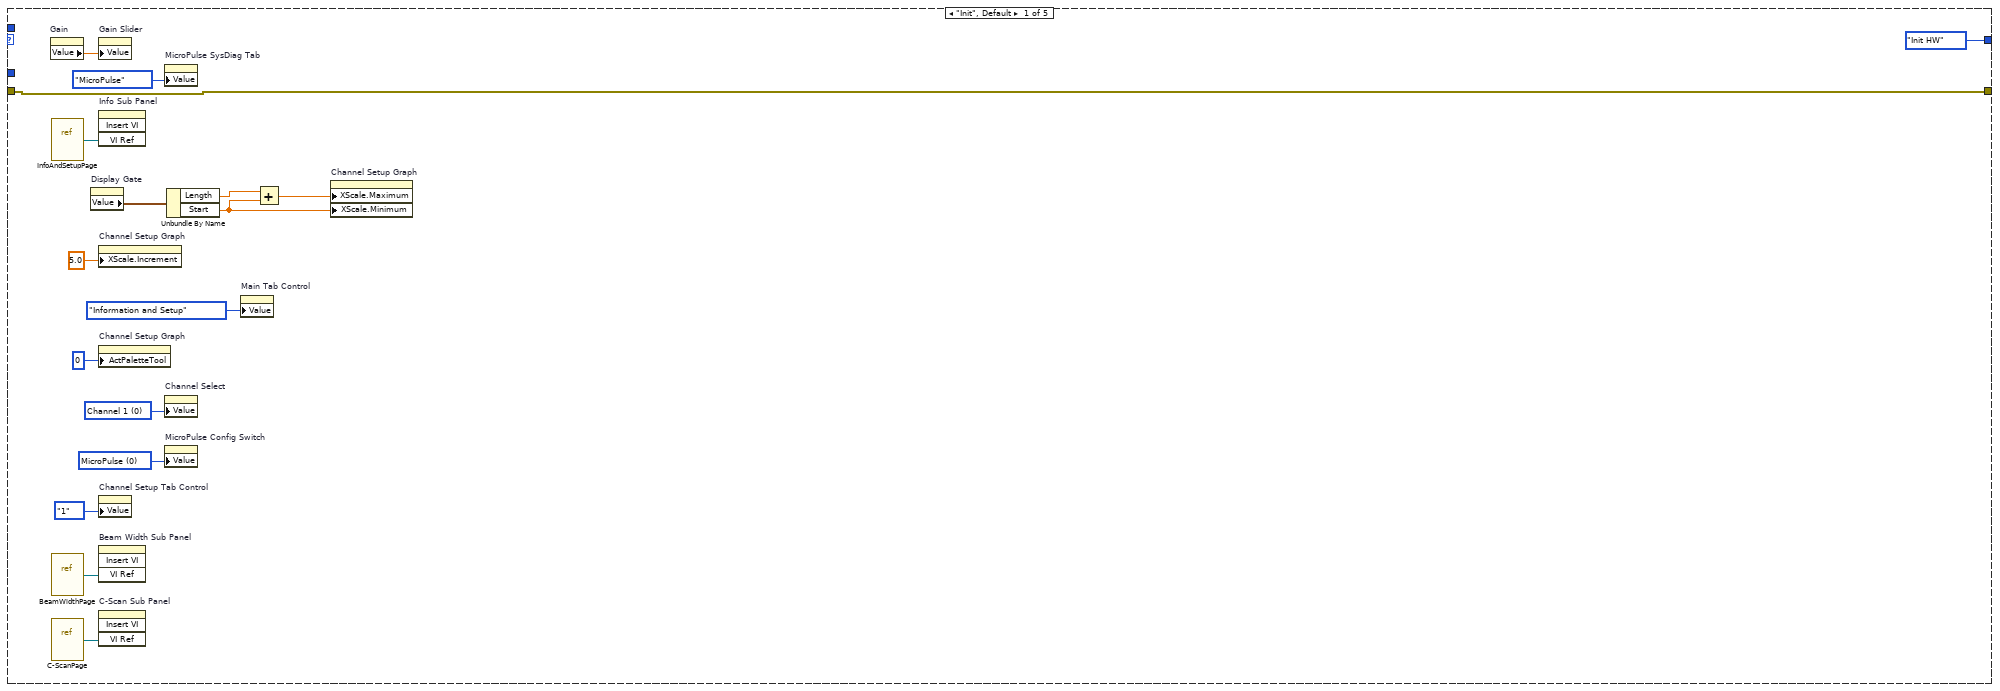
[diagram p2: hidden frame]
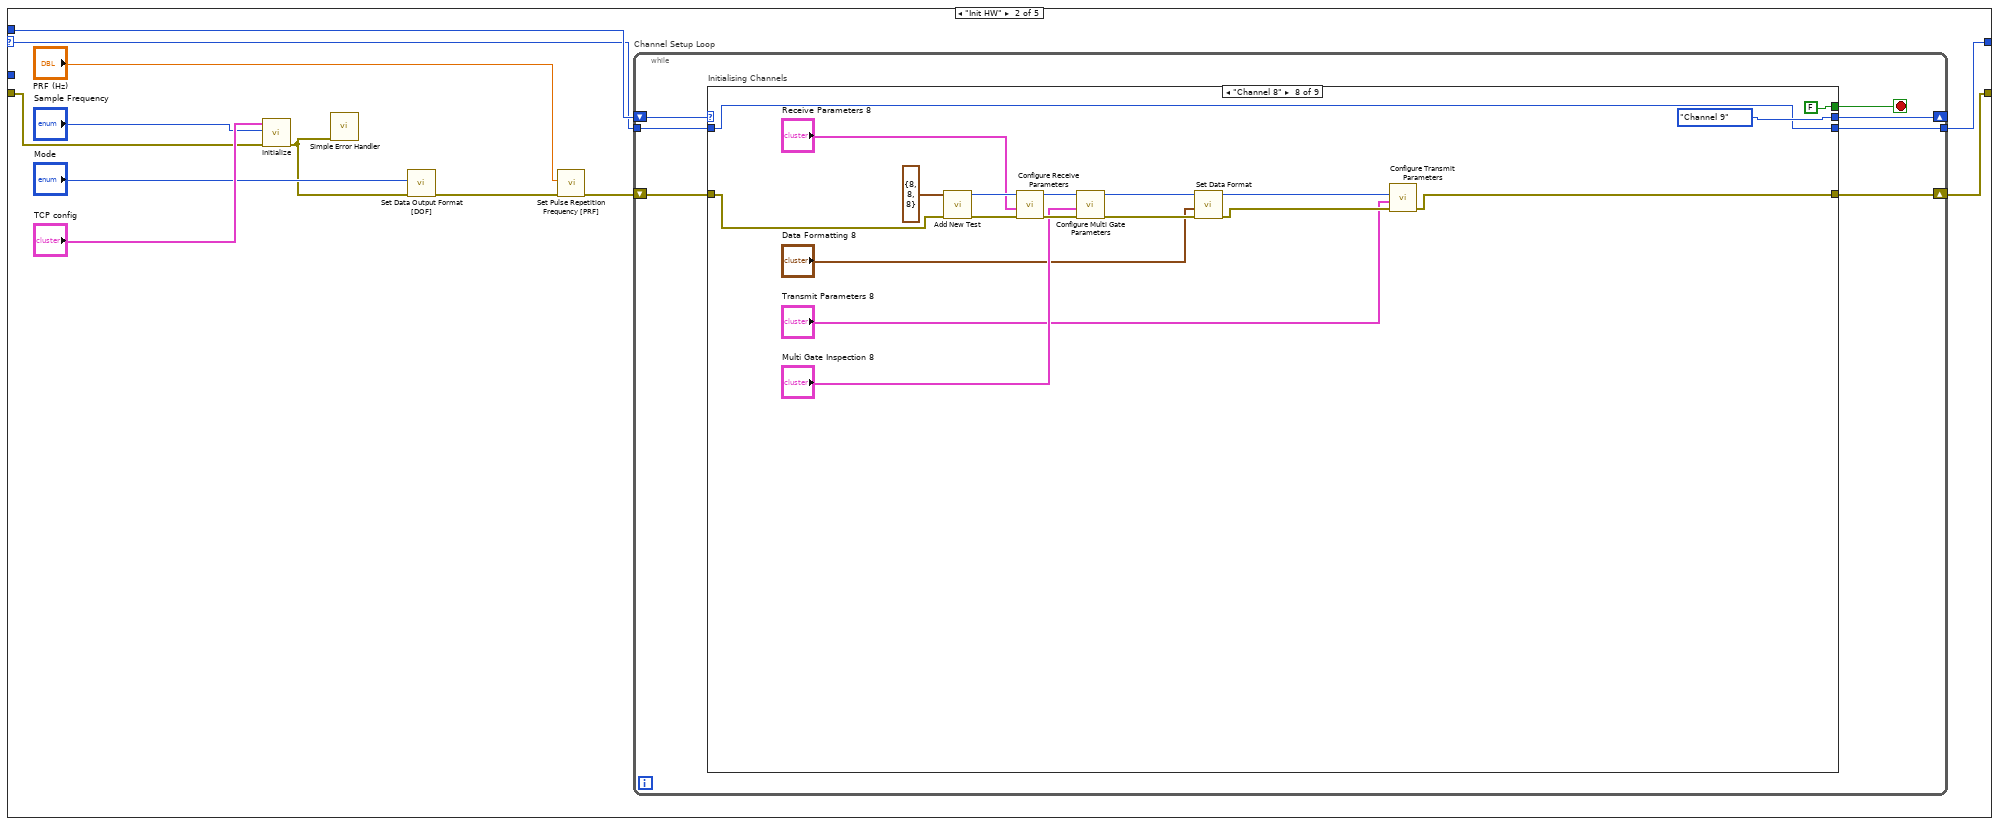
[diagram p3: hidden frame]
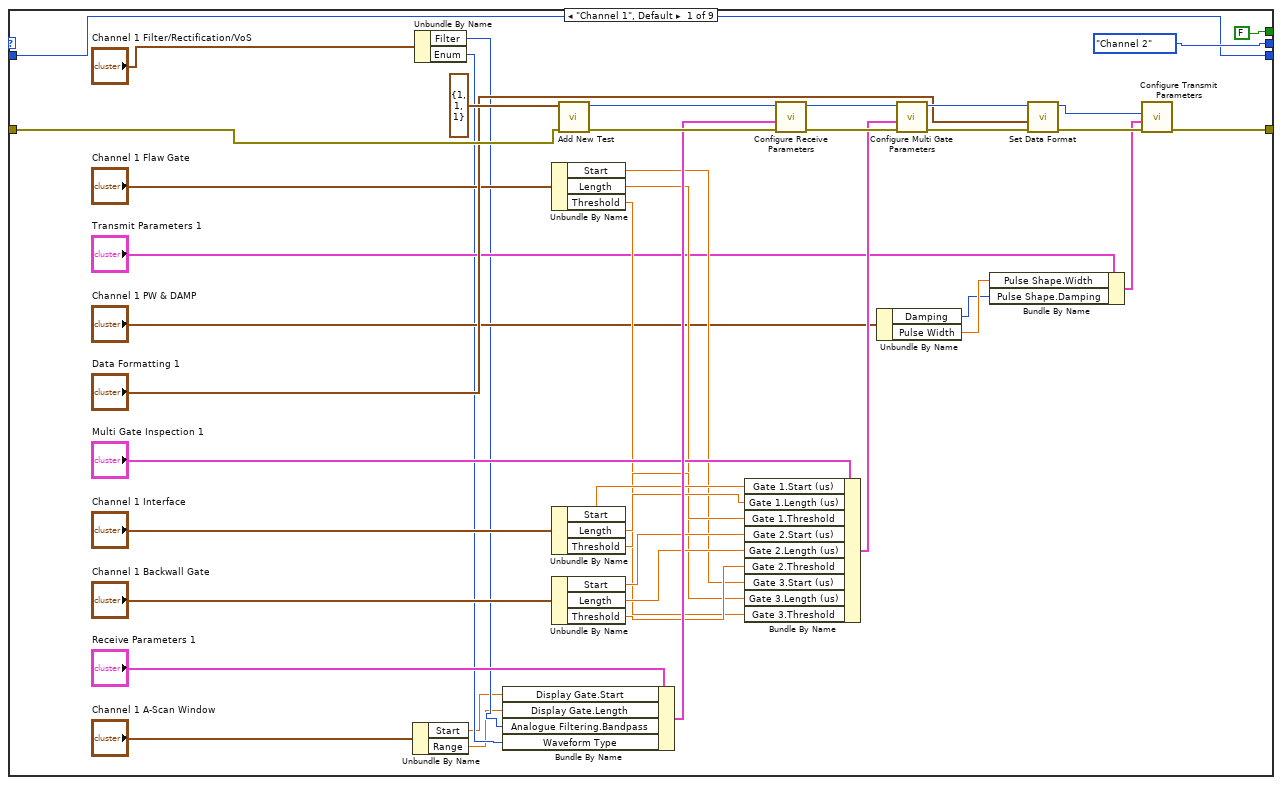
[diagram p4: hidden frame]
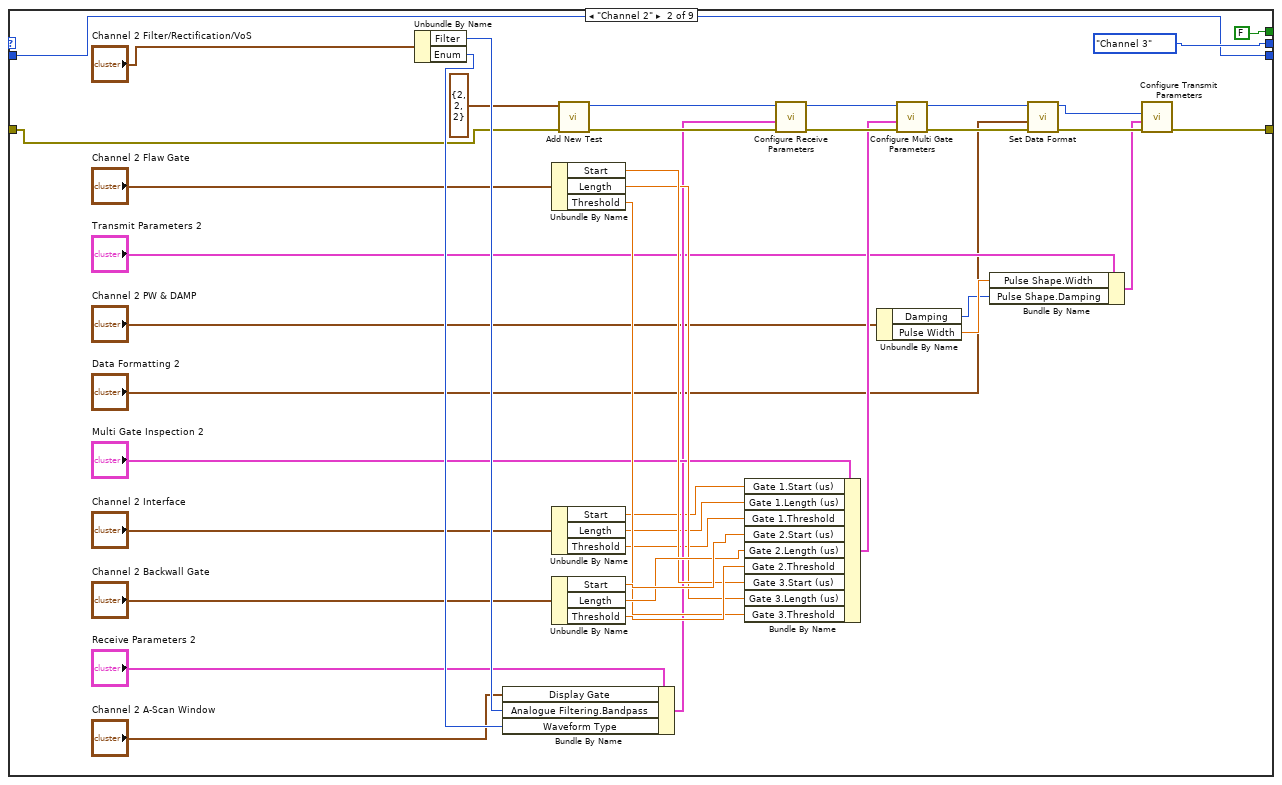
[diagram p5: hidden frame]
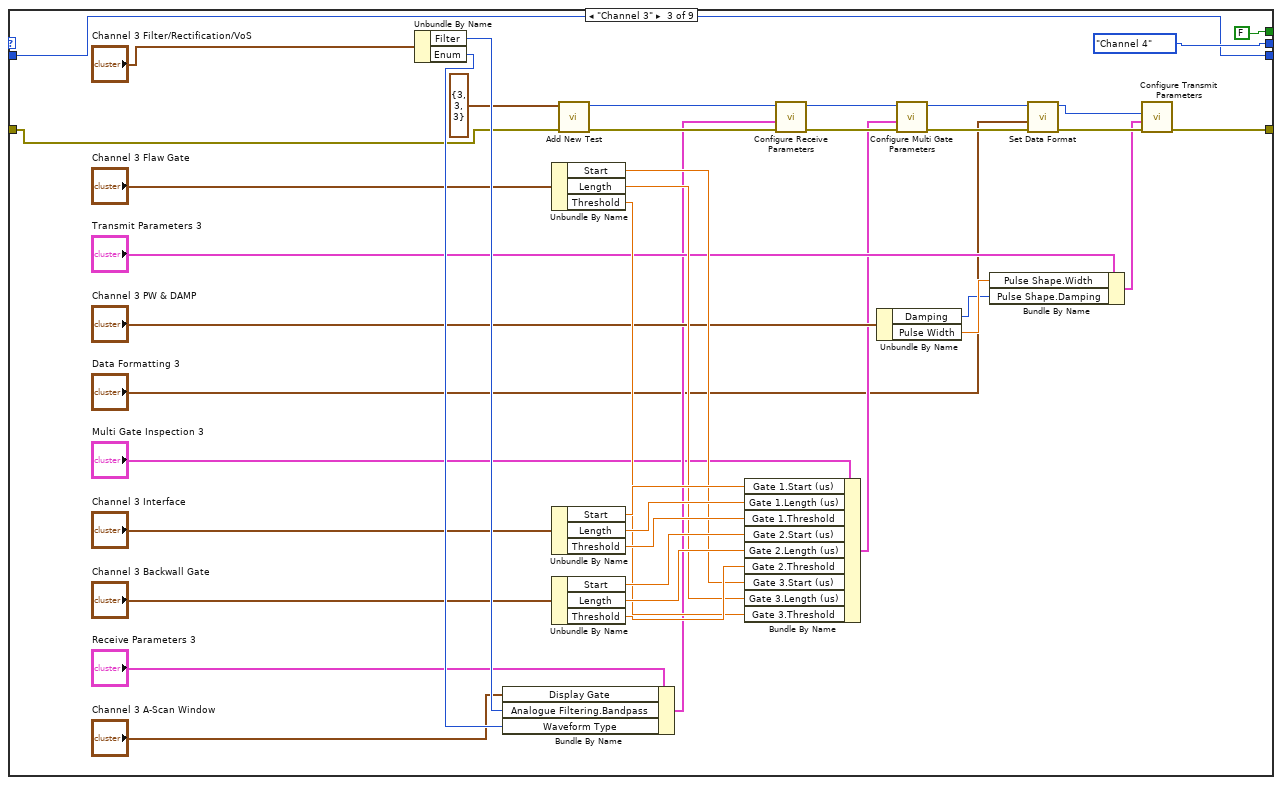
[diagram p6: hidden frame]
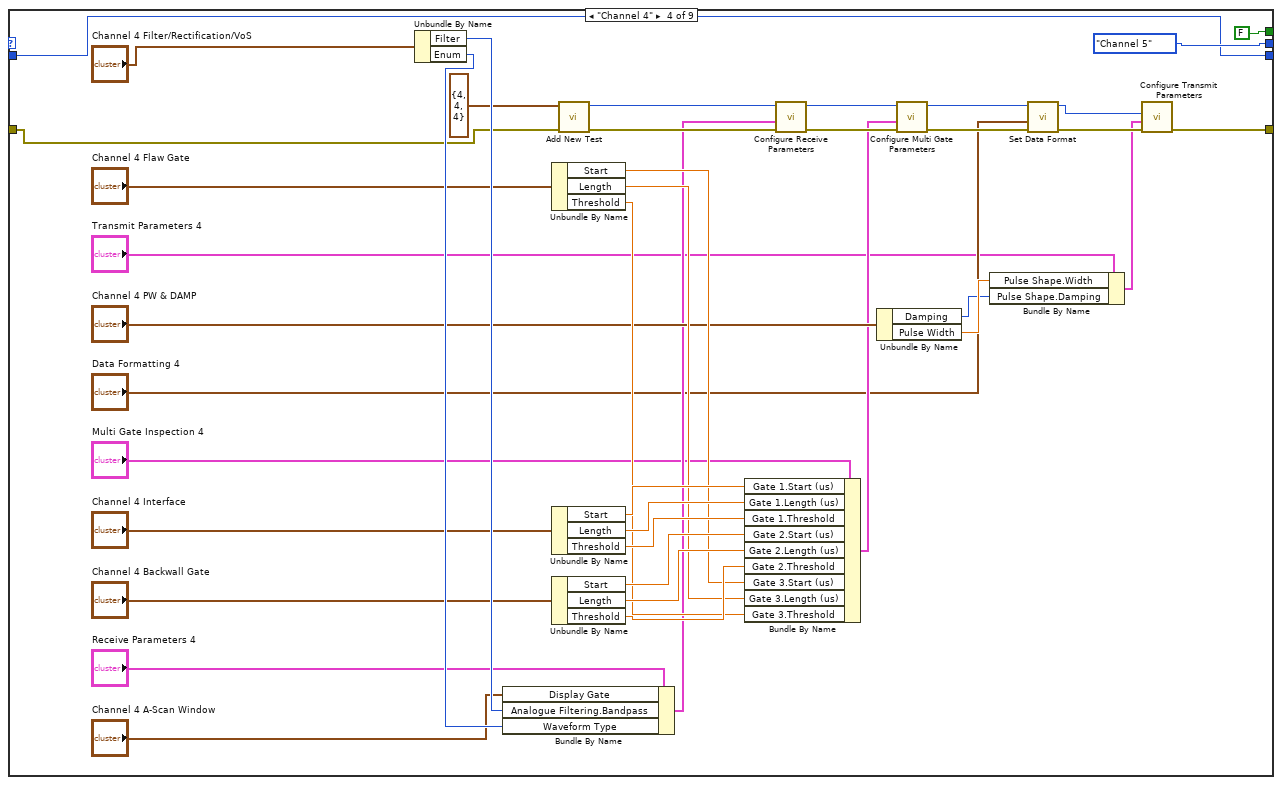
[diagram p7: hidden frame]
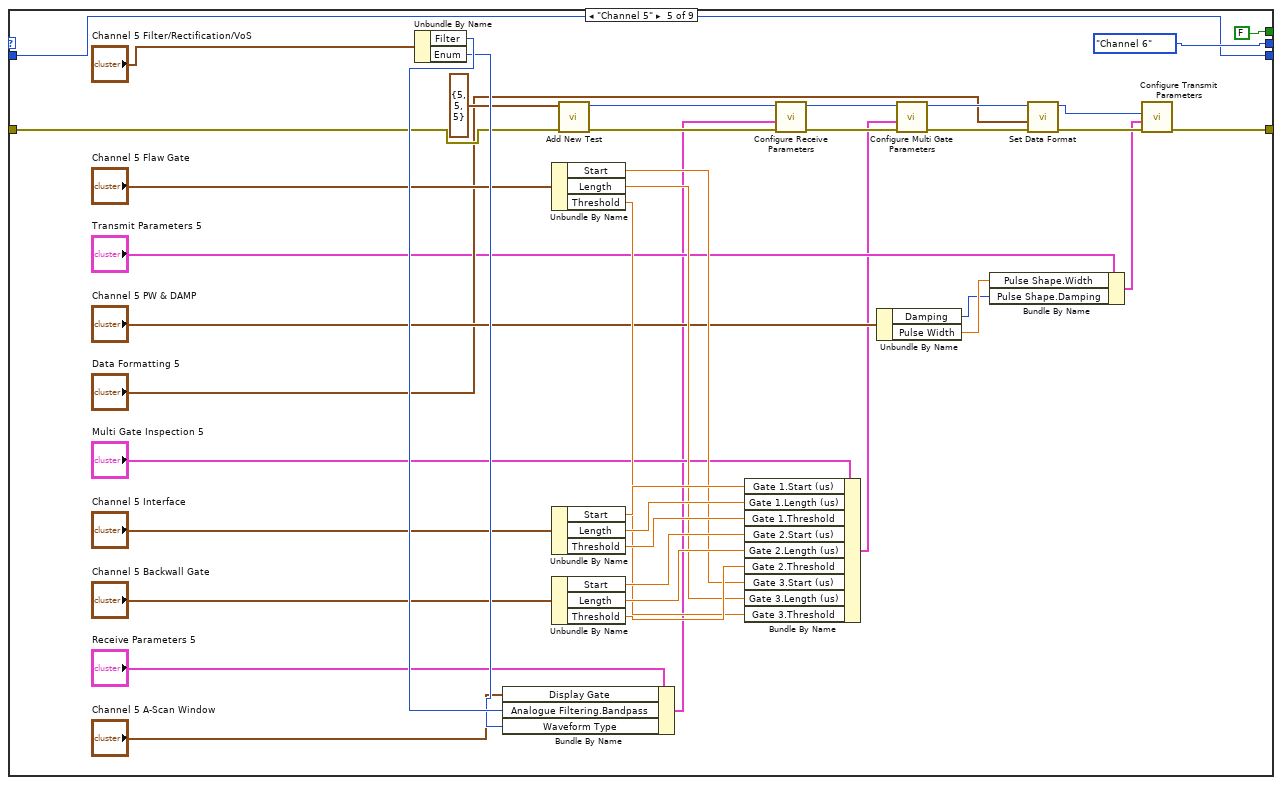
[diagram p8: hidden frame]
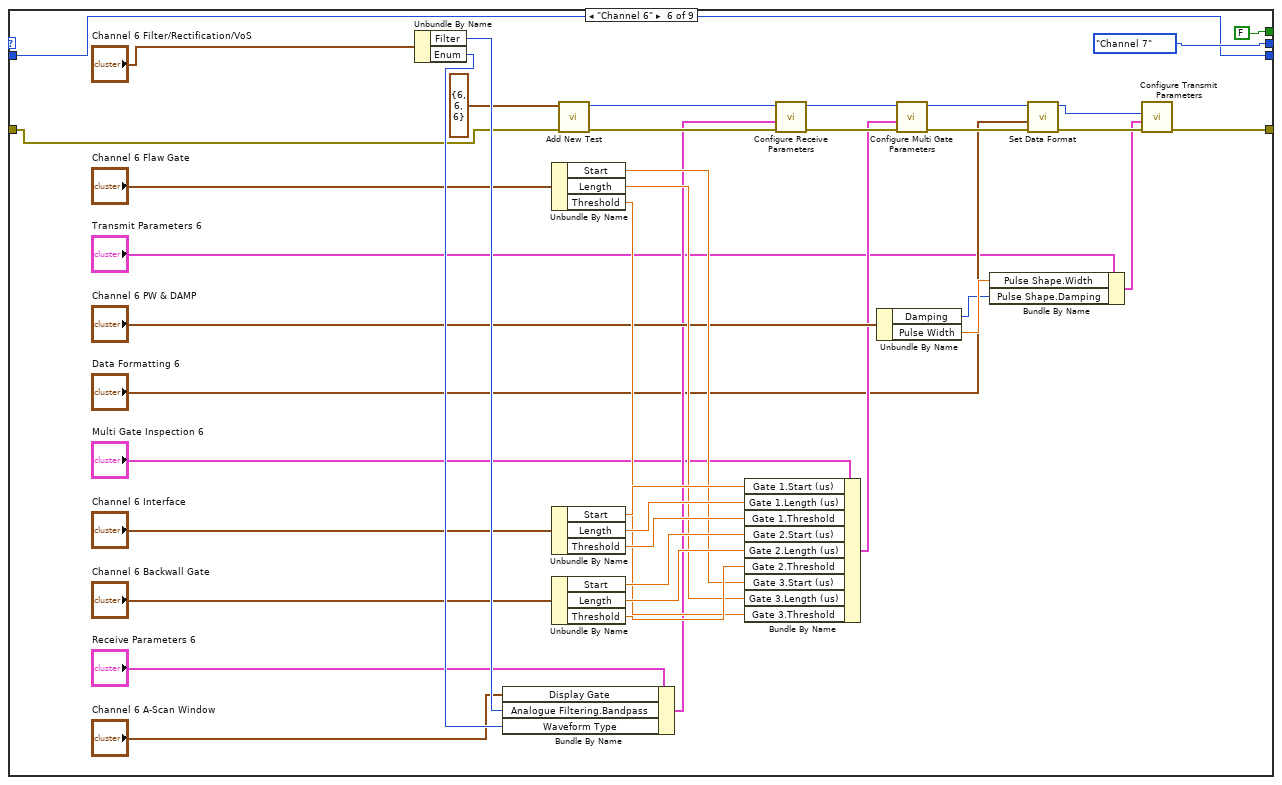
[diagram p9: hidden frame]
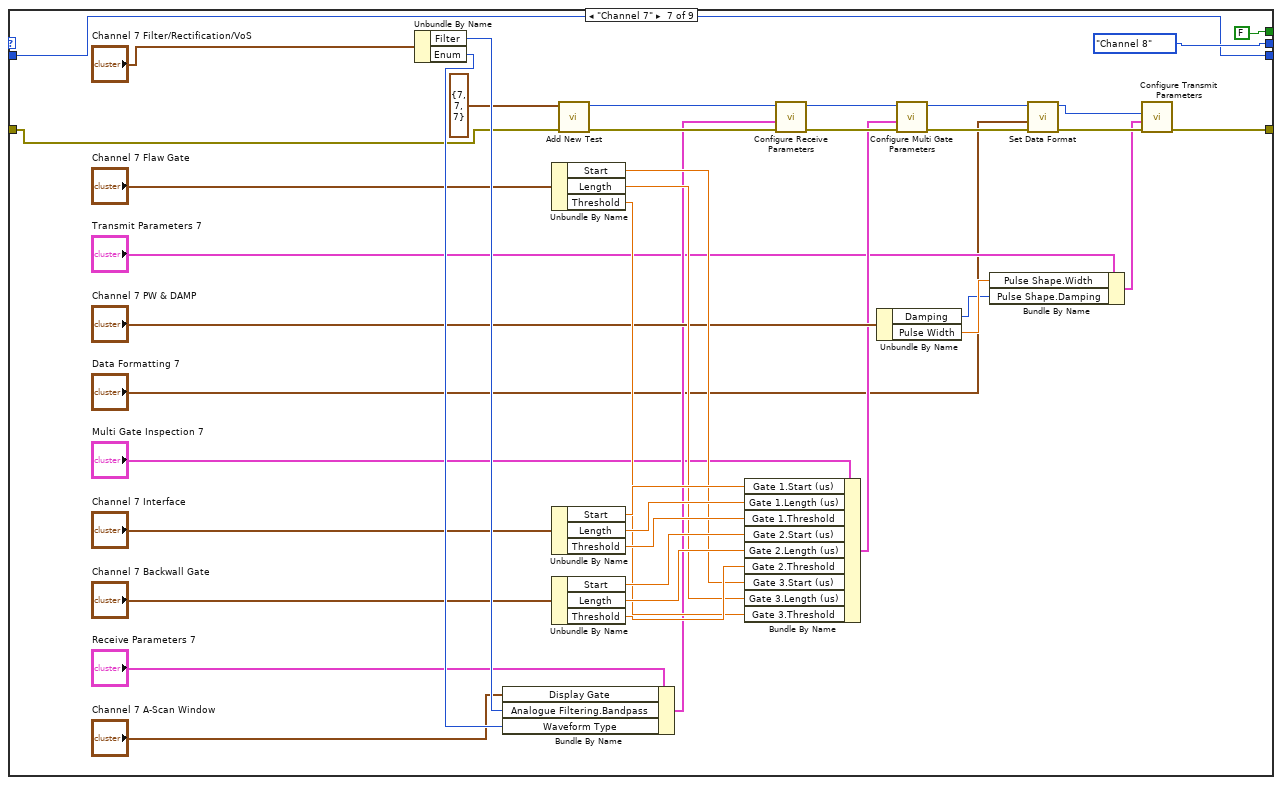
[diagram p10: hidden frame]
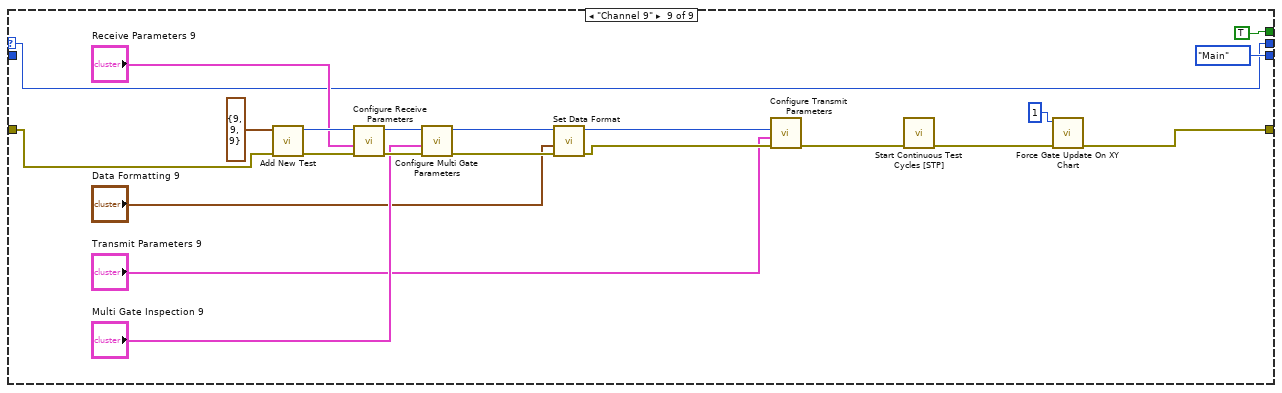
[diagram p11: hidden frame]
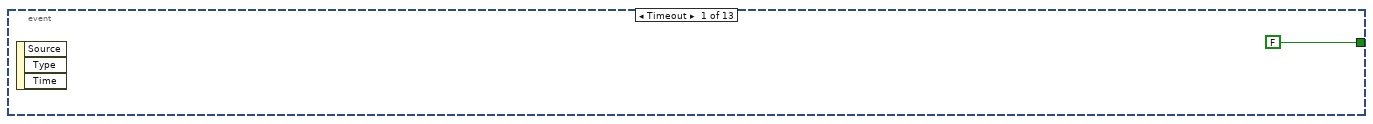
[diagram p13: hidden frame]
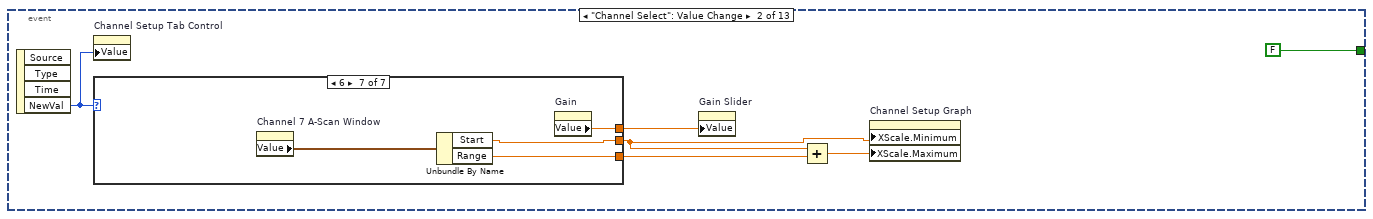
[diagram p14: hidden frame]
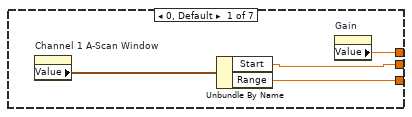
[diagram p15: hidden frame]
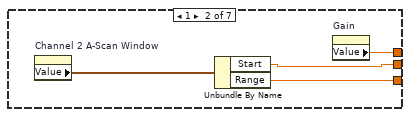
[diagram p16: hidden frame]
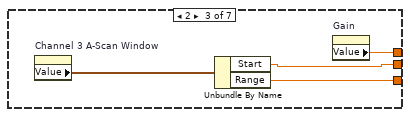
[diagram p17: hidden frame]
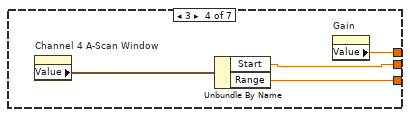
[diagram p18: hidden frame]
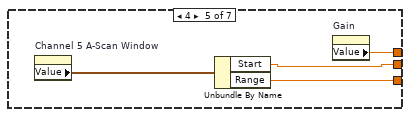
[diagram p19: hidden frame]
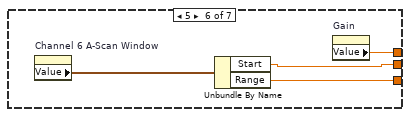
[diagram p20: hidden frame]
diagram:
  n1 = xnode "Error Ring"() -> ("error out"=w3:errorcluster)
  n2 = while {
    tunnel: T28."Channel 1" -> [w9]
    shift-right: [w8] -> _
    shift-left: T29."Init" -> [w10]
    shift-right: [w5] -> _
    shift-left: w3 -> [w6]
    stop <- "stop" stop-if-true
    n3 = property on="Main Tab Control" class="TabCtl (strict)"() -> ("Value"=w4:T1)  [unwired: 2 in, 2 out]
    n4 = case shown="\"Main\"" w10 {
      selector: w10 -> [_ w37 _ _ w624]
      tunnel: w9 -> [_ w39 _ _ _]
      tunnel: [T29."Init HW" w38 w369 T29."Shutdown" w624] -> w8
      tunnel: w6 -> [w26 w28 w374 w621 w623]
      tunnel: [w26 w34 w373 w621 w623] -> w5
      tunnel: w4 -> [_ _ w372 _ _]
      frame "Init", Default {
        w21 = u16 0 items=["MicroPulse", "Channel 1", "Channel 2", "Channel 3", "Channel 4", "Channel 5", "Channel 6", "Channel 7", "Channel 8", "Channel 9"] ("MicroPulse Config Switch")
        w22 = u16 0 items=["Channel 1", "Channel 2", "Channel 3", "Channel 4", "Channel 5", "Channel 6", "Channel 7", "Channel 8", "Channel 9"] ("Channel Select")
        n5 = property on="Gain" class="DigNum (strict)"() -> ("Value"=w16:dbl)  [unwired: 2 in, 2 out]
        n6 = vi-ref "InfoAndSetupPage.vi"() -> (w13:refnum<vi>)
        n7 = vi-ref "BeamWidthPage.vi"() -> (w12:refnum<vi>)
        n8 = vi-ref "C-ScanPage.vi"() -> (w11:refnum<vi>)
        n9 = property on="Display Gate" class="Clust (strict)"() -> ("Value"=w19:T13)  [unwired: 2 in, 2 out]
        n10 = property on="Gain Slider" class="Slide (strict)"("Value"=w16) -> ()  [unwired: 2 in, 2 out]
        n11 = invoke on="Info Sub Panel" class="SubPnl" method="Insert VI"("VI Ref"=w13) -> ()  [unwired: 3 in, 4 out]
        n12 = property on="Channel Setup Graph" class="XYGraph (strict)"("XScale.Increment"=5.0 ("X Scale.Range:Increment")) -> ()  [unwired: 2 in, 2 out]
        n13 = property on="Channel Setup Graph" class="XYGraph (strict)"("ActPaletteTool"=0 ("Palette:Active Tool")) -> ()  [unwired: 2 in, 2 out]
        n14 = property on="Channel Setup Tab Control" class="TabCtl (strict)"("Value"=enum32{"1", "2", "3", "4", "5", "6", "7"}."1" ("Channel Setup Tab Control")) -> ()  [unwired: 2 in, 2 out]
        n15 = invoke on="Beam Width Sub Panel" class="SubPnl" method="Insert VI"("VI Ref"=w12) -> ()  [unwired: 3 in, 4 out]
        n16 = invoke on="C-Scan Sub Panel" class="SubPnl" method="Insert VI"("VI Ref"=w11) -> ()  [unwired: 3 in, 4 out]
        n17 = property on="MicroPulse SysDiag Tab" class="TabCtl (strict)"("Value"=T8."MicroPulse" ("MicroPulse SysDiag Tab")) -> ()  [unwired: 2 in, 2 out]
        n18 = property on="Channel Select" class="Ring (strict)"("Value"=w22) -> ()  [unwired: 2 in, 2 out]
        n19 = property on="MicroPulse Config Switch" class="Ring (strict)"("Value"=w21) -> ()  [unwired: 2 in, 2 out]
        n20 = Unbundle By Name(w19) -> ("Length"=w17:dbl, "Start"=w15:dbl)
        n21 = property on="Main Tab Control" class="TabCtl (strict)"("Value"=T1."Information and Setup" ("Main Tab Control")) -> ()  [unwired: 2 in, 2 out]
        n22 = Add(x=w17, y=w15) -> (x+y=w18:dbl)
        n23 = property on="Channel Setup Graph" class="XYGraph (strict)"("XScale.Maximum"=w18, "XScale.Minimum"=w15) -> ()  [unwired: 2 in, 2 out]
      }
      frame "Init HW" {
        n24 = call <instrlib>:"Initialize.vi"("error in (no error)"=w28, "Sample Frequency"="Sample Frequency", "TCP config"="TCP config") -> ("error out"=w29:errorcluster)  [unwired: 7 in, 1 out]
        n25 = call <vilib>:"Simple Error Handler.vi"("error in (no error)"=w29) -> ()  [unwired: 4 in, 5 out]
        n26 = call <instrlib>:"Set Data Output Format [DOF].vi"("error in (no error)"=w29, "Mode"="Mode") -> ("error out"=w33:errorcluster)  [unwired: 8 in, 1 out]
        n27 = call <instrlib>:"Set Pulse Repetition Frequency [PRF].vi"("error in (no error)"=w33, "Frequency (Hz)"="PRF (Hz)") -> ("error out"=w32:errorcluster)  [unwired: 8 in, 1 out]
        n28 = while "Channel Setup Loop" {
          shift-right: [w44] -> w34
          shift-left: w32 -> [w45]
          shift-right: [w43] -> _
          shift-left: w39 -> [w46]
          tunnel: [w41] -> w38
          tunnel: w37 -> [w40]
          stop <- w42 stop-if-true
          n29 = case "Initialising Channels" shown="\"Channel 8\"" w46 {
            selector: w46 -> [_ _ _ _ _ _ _ _ w351]
            tunnel: w45 -> [w88 w94 w130 w170 w216 w258 w299 w339 w360]
            tunnel: [w81 w95 w131 w171 w224 w249 w292 w338 w348] -> w44
            tunnel: [T28."Channel 2" T28."Channel 3" T28."Channel 4" T28."Channel 5" T28."Channel 6" T28."Channel 7" T28."Channel 8" T28."Channel 9" w351] -> w43
            tunnel: [FALSE FALSE FALSE FALSE FALSE FALSE FALSE FALSE TRUE] -> w42
            tunnel: [w75 w127 w167 w207 w247 w287 w327 w330 T29."Main"] -> w41
            tunnel: w40 -> [w75 w127 w167 w207 w247 w287 w327 w330 _]
            frame "Channel 1", Default {
              n30 = Unbundle By Name("Channel 1 A-Scan Window") -> ("Start"=w48:dbl, "Range"=w47:dbl)
              n31 = Unbundle By Name("Channel 1 Filter/Rectification/VoS") -> ("Filter"=w51:T4, "Enum"=w50:T31)
              n32 = Bundle By Name(cluster="Receive Parameters 1", "Display Gate.Start"=w48, "Display Gate.Length"=w47, "Analogue Filtering.Bandpass"=w51, "Waveform Type"=w50) -> (w72:T12)
              n33 = Unbundle By Name("Channel 1 Flaw Gate") -> ("Start"=w61:dbl, "Length"=w60:dbl, "Threshold"=w59:dbl)
              n34 = Unbundle By Name("Channel 1 Interface") -> ("Start"=w69:dbl, "Length"=w68:dbl, "Threshold"=w67:dbl)
              n35 = Unbundle By Name("Channel 1 Backwall Gate") -> ("Start"=w65:dbl, "Length"=w64:dbl, "Threshold"=w63:dbl)
              n36 = call <instrlib>:"Add New Test.vi"("error in (no error)"=w88, "Test Parameters"=T30 {"Test No."=1, "Tx Channel"=1, "Rx Channel"=1}) -> ("error out"=w80:errorcluster, "Test No. out"=w77:u32)  [unwired: 6 in, 2 out]
              n37 = Bundle By Name(cluster="Multi Gate Inspection 1", "Gate 1.Start (us)"=w69, "Gate 1.Length (us)"=w68, "Gate 1.Threshold"=w67, "Gate 2.Start (us)"=w65, "Gate 2.Length (us)"=w64, "Gate 2.Threshold"=w63, "Gate 3.Start (us)"=w61, "Gate 3.Length (us)"=w60, "Gate 3.Threshold"=w59) -> (w58:T19)
              n38 = call <instrlib>:"Configure Receive Parameters.vi"("error in (no error)"=w80, "Receive Parameters"=w72, "Test No."=w77) -> ("error out"=w86:errorcluster, "Test No. out"=w85:u32)  [unwired: 6 in, 1 out]
              n39 = Unbundle By Name("Channel 1 PW & DAMP") -> ("Damping"=w52:T7, "Pulse Width"=w53:dbl)
              n40 = call <instrlib>:"Configure Multi Gate Parameters.vi"("error in (no error)"=w86, "Multi Gate Inspection"=w58, "Test Number"=w85) -> ("error out"=w82:errorcluster, "Test Number out"=w78:u32)  [unwired: 6 in, 1 out]
              n41 = Bundle By Name(cluster="Transmit Parameters 1", "Pulse Shape.Width"=w53, "Pulse Shape.Damping"=w52) -> (w54:T26)
              n42 = call <instrlib>:"Set Data Format.vi"("error in (no error)"=w82, "Data Formatting"="Data Formatting 1", "Test No."=w78) -> ("error out"=w84:errorcluster, "Test No. out"=w83:u32)  [unwired: 6 in, 1 out]
              n43 = call <instrlib>:"Configure Transmit Parameters.vi"("error in (no error)"=w84, "Transmit Parameters"=w54, "Tx Channel"=w83) -> ("error out"=w81:errorcluster)  [unwired: 7 in, 1 out]
            }
            frame "Channel 2" {
              n44 = Unbundle By Name("Channel 2 Filter/Rectification/VoS") -> ("Filter"=w110:T4, "Enum"=w109:T31)
              n45 = Bundle By Name(cluster="Receive Parameters 2", "Display Gate"="Channel 2 A-Scan Window", "Analogue Filtering.Bandpass"=w110, "Waveform Type"=w109) -> (w103:T12)
              n46 = Unbundle By Name("Channel 2 Flaw Gate") -> ("Start"=w114:dbl, "Length"=w113:dbl, "Threshold"=w112:dbl)
              n47 = Unbundle By Name("Channel 2 Interface") -> ("Start"=w92:dbl, "Length"=w91:dbl, "Threshold"=w90:dbl)
              n48 = Unbundle By Name("Channel 2 Backwall Gate") -> ("Start"=w117:dbl, "Length"=w116:dbl, "Threshold"=w115:dbl)
              n49 = call <instrlib>:"Add New Test.vi"("error in (no error)"=w94, "Test Parameters"=T30 {"Test No."=2, "Tx Channel"=2, "Rx Channel"=2}) -> ("error out"=w120:errorcluster, "Test No. out"=w118:u32)  [unwired: 6 in, 2 out]
              n50 = Bundle By Name(cluster="Multi Gate Inspection 2", "Gate 1.Start (us)"=w92, "Gate 1.Length (us)"=w91, "Gate 1.Threshold"=w90, "Gate 2.Start (us)"=w117, "Gate 2.Length (us)"=w116, "Gate 2.Threshold"=w115, "Gate 3.Start (us)"=w114, "Gate 3.Length (us)"=w113, "Gate 3.Threshold"=w112) -> (w111:T19)
              n51 = call <instrlib>:"Configure Receive Parameters.vi"("error in (no error)"=w120, "Receive Parameters"=w103, "Test No."=w118) -> ("error out"=w125:errorcluster, "Test No. out"=w124:u32)  [unwired: 6 in, 1 out]
              n52 = Unbundle By Name("Channel 2 PW & DAMP") -> ("Damping"=w107:T7, "Pulse Width"=w108:dbl)
              n53 = call <instrlib>:"Configure Multi Gate Parameters.vi"("error in (no error)"=w125, "Multi Gate Inspection"=w111, "Test Number"=w124) -> ("error out"=w121:errorcluster, "Test Number out"=w119:u32)  [unwired: 6 in, 1 out]
              n54 = Bundle By Name(cluster="Transmit Parameters 2", "Pulse Shape.Width"=w108, "Pulse Shape.Damping"=w107) -> (w89:T26)
              n55 = call <instrlib>:"Set Data Format.vi"("error in (no error)"=w121, "Data Formatting"="Data Formatting 2", "Test No."=w119) -> ("error out"=w123:errorcluster, "Test No. out"=w122:u32)  [unwired: 6 in, 1 out]
              n56 = call <instrlib>:"Configure Transmit Parameters.vi"("error in (no error)"=w123, "Transmit Parameters"=w89, "Tx Channel"=w122) -> ("error out"=w95:errorcluster)  [unwired: 7 in, 1 out]
            }
            frame "Channel 3" {
              n57 = Unbundle By Name("Channel 3 Filter/Rectification/VoS") -> ("Filter"=w148:T4, "Enum"=w147:T31)
              n58 = Bundle By Name(cluster="Receive Parameters 3", "Display Gate"="Channel 3 A-Scan Window", "Analogue Filtering.Bandpass"=w148, "Waveform Type"=w147) -> (w135:T12)
              n59 = Unbundle By Name("Channel 3 Flaw Gate") -> ("Start"=w151:dbl, "Length"=w150:dbl, "Threshold"=w149:dbl)
              n60 = Unbundle By Name("Channel 3 Interface") -> ("Start"=w157:dbl, "Length"=w156:dbl, "Threshold"=w155:dbl)
              n61 = Unbundle By Name("Channel 3 Backwall Gate") -> ("Start"=w154:dbl, "Length"=w153:dbl, "Threshold"=w152:dbl)
              n62 = call <instrlib>:"Add New Test.vi"("error in (no error)"=w130, "Test Parameters"=T30 {"Test No."=3, "Tx Channel"=3, "Rx Channel"=3}) -> ("error out"=w160:errorcluster, "Test No. out"=w158:u32)  [unwired: 6 in, 2 out]
              n63 = Bundle By Name(cluster="Multi Gate Inspection 3", "Gate 1.Start (us)"=w157, "Gate 1.Length (us)"=w156, "Gate 1.Threshold"=w155, "Gate 2.Start (us)"=w154, "Gate 2.Length (us)"=w153, "Gate 2.Threshold"=w152, "Gate 3.Start (us)"=w151, "Gate 3.Length (us)"=w150, "Gate 3.Threshold"=w149) -> (w133:T19)
              n64 = call <instrlib>:"Configure Receive Parameters.vi"("error in (no error)"=w160, "Receive Parameters"=w135, "Test No."=w158) -> ("error out"=w165:errorcluster, "Test No. out"=w164:u32)  [unwired: 6 in, 1 out]
              n65 = Unbundle By Name("Channel 3 PW & DAMP") -> ("Damping"=w145:T7, "Pulse Width"=w146:dbl)
              n66 = call <instrlib>:"Configure Multi Gate Parameters.vi"("error in (no error)"=w165, "Multi Gate Inspection"=w133, "Test Number"=w164) -> ("error out"=w161:errorcluster, "Test Number out"=w159:u32)  [unwired: 6 in, 1 out]
              n67 = Bundle By Name(cluster="Transmit Parameters 3", "Pulse Shape.Width"=w146, "Pulse Shape.Damping"=w145) -> (w138:T26)
              n68 = call <instrlib>:"Set Data Format.vi"("error in (no error)"=w161, "Data Formatting"="Data Formatting 3", "Test No."=w159) -> ("error out"=w163:errorcluster, "Test No. out"=w162:u32)  [unwired: 6 in, 1 out]
              n69 = call <instrlib>:"Configure Transmit Parameters.vi"("error in (no error)"=w163, "Transmit Parameters"=w138, "Tx Channel"=w162) -> ("error out"=w131:errorcluster)  [unwired: 7 in, 1 out]
            }
            frame "Channel 4" {
              n70 = Unbundle By Name("Channel 4 Filter/Rectification/VoS") -> ("Filter"=w188:T4, "Enum"=w187:T31)
              n71 = Bundle By Name(cluster="Receive Parameters 4", "Display Gate"="Channel 4 A-Scan Window", "Analogue Filtering.Bandpass"=w188, "Waveform Type"=w187) -> (w180:T12)
              n72 = Unbundle By Name("Channel 4 Flaw Gate") -> ("Start"=w191:dbl, "Length"=w190:dbl, "Threshold"=w189:dbl)
              n73 = Unbundle By Name("Channel 4 Interface") -> ("Start"=w197:dbl, "Length"=w196:dbl, "Threshold"=w195:dbl)
              n74 = Unbundle By Name("Channel 4 Backwall Gate") -> ("Start"=w194:dbl, "Length"=w193:dbl, "Threshold"=w192:dbl)
              n75 = call <instrlib>:"Add New Test.vi"("error in (no error)"=w170, "Test Parameters"=T30 {"Test No."=4, "Tx Channel"=4, "Rx Channel"=4}) -> ("error out"=w200:errorcluster, "Test No. out"=w198:u32)  [unwired: 6 in, 2 out]
              n76 = Bundle By Name(cluster="Multi Gate Inspection 4", "Gate 1.Start (us)"=w197, "Gate 1.Length (us)"=w196, "Gate 1.Threshold"=w195, "Gate 2.Start (us)"=w194, "Gate 2.Length (us)"=w193, "Gate 2.Threshold"=w192, "Gate 3.Start (us)"=w191, "Gate 3.Length (us)"=w190, "Gate 3.Threshold"=w189) -> (w175:T19)
              n77 = call <instrlib>:"Configure Receive Parameters.vi"("error in (no error)"=w200, "Receive Parameters"=w180, "Test No."=w198) -> ("error out"=w205:errorcluster, "Test No. out"=w204:u32)  [unwired: 6 in, 1 out]
              n78 = Unbundle By Name("Channel 4 PW & DAMP") -> ("Damping"=w185:T7, "Pulse Width"=w186:dbl)
              n79 = call <instrlib>:"Configure Multi Gate Parameters.vi"("error in (no error)"=w205, "Multi Gate Inspection"=w175, "Test Number"=w204) -> ("error out"=w201:errorcluster, "Test Number out"=w199:u32)  [unwired: 6 in, 1 out]
              n80 = Bundle By Name(cluster="Transmit Parameters 4", "Pulse Shape.Width"=w186, "Pulse Shape.Damping"=w185) -> (w172:T26)
              n81 = call <instrlib>:"Set Data Format.vi"("error in (no error)"=w201, "Data Formatting"="Data Formatting 4", "Test No."=w199) -> ("error out"=w203:errorcluster, "Test No. out"=w202:u32)  [unwired: 6 in, 1 out]
              n82 = call <instrlib>:"Configure Transmit Parameters.vi"("error in (no error)"=w203, "Transmit Parameters"=w172, "Tx Channel"=w202) -> ("error out"=w171:errorcluster)  [unwired: 7 in, 1 out]
            }
            frame "Channel 5" {
              n83 = Unbundle By Name("Channel 5 Filter/Rectification/VoS") -> ("Filter"=w228:T4, "Enum"=w227:T31)
              n84 = Bundle By Name(cluster="Receive Parameters 5", "Display Gate"="Channel 5 A-Scan Window", "Analogue Filtering.Bandpass"=w228, "Waveform Type"=w227) -> (w209:T12)
              n85 = Unbundle By Name("Channel 5 Flaw Gate") -> ("Start"=w231:dbl, "Length"=w230:dbl, "Threshold"=w229:dbl)
              n86 = Unbundle By Name("Channel 5 Interface") -> ("Start"=w237:dbl, "Length"=w236:dbl, "Threshold"=w235:dbl)
              n87 = Unbundle By Name("Channel 5 Backwall Gate") -> ("Start"=w234:dbl, "Length"=w233:dbl, "Threshold"=w232:dbl)
              n88 = call <instrlib>:"Add New Test.vi"("error in (no error)"=w216, "Test Parameters"=T30 {"Test No."=5, "Tx Channel"=5, "Rx Channel"=5}) -> ("error out"=w240:errorcluster, "Test No. out"=w238:u32)  [unwired: 6 in, 2 out]
              n89 = Bundle By Name(cluster="Multi Gate Inspection 5", "Gate 1.Start (us)"=w237, "Gate 1.Length (us)"=w236, "Gate 1.Threshold"=w235, "Gate 2.Start (us)"=w234, "Gate 2.Length (us)"=w233, "Gate 2.Threshold"=w232, "Gate 3.Start (us)"=w231, "Gate 3.Length (us)"=w230, "Gate 3.Threshold"=w229) -> (w210:T19)
              n90 = call <instrlib>:"Configure Receive Parameters.vi"("error in (no error)"=w240, "Receive Parameters"=w209, "Test No."=w238) -> ("error out"=w245:errorcluster, "Test No. out"=w244:u32)  [unwired: 6 in, 1 out]
              n91 = Unbundle By Name("Channel 5 PW & DAMP") -> ("Damping"=w225:T7, "Pulse Width"=w226:dbl)
              n92 = call <instrlib>:"Configure Multi Gate Parameters.vi"("error in (no error)"=w245, "Multi Gate Inspection"=w210, "Test Number"=w244) -> ("error out"=w241:errorcluster, "Test Number out"=w239:u32)  [unwired: 6 in, 1 out]
              n93 = Bundle By Name(cluster="Transmit Parameters 5", "Pulse Shape.Width"=w226, "Pulse Shape.Damping"=w225) -> (w211:T26)
              n94 = call <instrlib>:"Set Data Format.vi"("error in (no error)"=w241, "Data Formatting"="Data Formatting 5", "Test No."=w239) -> ("error out"=w243:errorcluster, "Test No. out"=w242:u32)  [unwired: 6 in, 1 out]
              n95 = call <instrlib>:"Configure Transmit Parameters.vi"("error in (no error)"=w243, "Transmit Parameters"=w211, "Tx Channel"=w242) -> ("error out"=w224:errorcluster)  [unwired: 7 in, 1 out]
            }
            frame "Channel 6" {
              n96 = Unbundle By Name("Channel 6 Filter/Rectification/VoS") -> ("Filter"=w268:T4, "Enum"=w267:T31)
              n97 = Bundle By Name(cluster="Receive Parameters 6", "Display Gate"="Channel 6 A-Scan Window", "Analogue Filtering.Bandpass"=w268, "Waveform Type"=w267) -> (w255:T12)
              n98 = Unbundle By Name("Channel 6 Flaw Gate") -> ("Start"=w271:dbl, "Length"=w270:dbl, "Threshold"=w269:dbl)
              n99 = Unbundle By Name("Channel 6 Interface") -> ("Start"=w277:dbl, "Length"=w276:dbl, "Threshold"=w275:dbl)
              n100 = Unbundle By Name("Channel 6 Backwall Gate") -> ("Start"=w274:dbl, "Length"=w273:dbl, "Threshold"=w272:dbl)
              n101 = call <instrlib>:"Add New Test.vi"("error in (no error)"=w258, "Test Parameters"=T30 {"Test No."=6, "Tx Channel"=6, "Rx Channel"=6}) -> ("error out"=w280:errorcluster, "Test No. out"=w278:u32)  [unwired: 6 in, 2 out]
              n102 = Bundle By Name(cluster="Multi Gate Inspection 6", "Gate 1.Start (us)"=w277, "Gate 1.Length (us)"=w276, "Gate 1.Threshold"=w275, "Gate 2.Start (us)"=w274, "Gate 2.Length (us)"=w273, "Gate 2.Threshold"=w272, "Gate 3.Start (us)"=w271, "Gate 3.Length (us)"=w270, "Gate 3.Threshold"=w269) -> (w253:T19)
              n103 = call <instrlib>:"Configure Receive Parameters.vi"("error in (no error)"=w280, "Receive Parameters"=w255, "Test No."=w278) -> ("error out"=w285:errorcluster, "Test No. out"=w284:u32)  [unwired: 6 in, 1 out]
              n104 = Unbundle By Name("Channel 6 PW & DAMP") -> ("Damping"=w265:T7, "Pulse Width"=w266:dbl)
              n105 = call <instrlib>:"Configure Multi Gate Parameters.vi"("error in (no error)"=w285, "Multi Gate Inspection"=w253, "Test Number"=w284) -> ("error out"=w281:errorcluster, "Test Number out"=w279:u32)  [unwired: 6 in, 1 out]
              n106 = Bundle By Name(cluster="Transmit Parameters 6", "Pulse Shape.Width"=w266, "Pulse Shape.Damping"=w265) -> (w250:T26)
              n107 = call <instrlib>:"Set Data Format.vi"("error in (no error)"=w281, "Data Formatting"="Data Formatting 6", "Test No."=w279) -> ("error out"=w283:errorcluster, "Test No. out"=w282:u32)  [unwired: 6 in, 1 out]
              n108 = call <instrlib>:"Configure Transmit Parameters.vi"("error in (no error)"=w283, "Transmit Parameters"=w250, "Tx Channel"=w282) -> ("error out"=w249:errorcluster)  [unwired: 7 in, 1 out]
            }
            frame "Channel 7" {
              n109 = Unbundle By Name("Channel 7 Filter/Rectification/VoS") -> ("Filter"=w308:T4, "Enum"=w307:T31)
              n110 = Bundle By Name(cluster="Receive Parameters 7", "Display Gate"="Channel 7 A-Scan Window", "Analogue Filtering.Bandpass"=w308, "Waveform Type"=w307) -> (w300:T12)
              n111 = Unbundle By Name("Channel 7 Flaw Gate") -> ("Start"=w311:dbl, "Length"=w310:dbl, "Threshold"=w309:dbl)
              n112 = Unbundle By Name("Channel 7 Interface") -> ("Start"=w317:dbl, "Length"=w316:dbl, "Threshold"=w315:dbl)
              n113 = Unbundle By Name("Channel 7 Backwall Gate") -> ("Start"=w314:dbl, "Length"=w313:dbl, "Threshold"=w312:dbl)
              n114 = call <instrlib>:"Add New Test.vi"("error in (no error)"=w299, "Test Parameters"=T30 {"Test No."=7, "Tx Channel"=7, "Rx Channel"=7}) -> ("error out"=w320:errorcluster, "Test No. out"=w318:u32)  [unwired: 6 in, 2 out]
              n115 = Bundle By Name(cluster="Multi Gate Inspection 7", "Gate 1.Start (us)"=w317, "Gate 1.Length (us)"=w316, "Gate 1.Threshold"=w315, "Gate 2.Start (us)"=w314, "Gate 2.Length (us)"=w313, "Gate 2.Threshold"=w312, "Gate 3.Start (us)"=w311, "Gate 3.Length (us)"=w310, "Gate 3.Threshold"=w309) -> (w296:T19)
              n116 = call <instrlib>:"Configure Receive Parameters.vi"("error in (no error)"=w320, "Receive Parameters"=w300, "Test No."=w318) -> ("error out"=w325:errorcluster, "Test No. out"=w324:u32)  [unwired: 6 in, 1 out]
              n117 = Unbundle By Name("Channel 7 PW & DAMP") -> ("Damping"=w305:T7, "Pulse Width"=w306:dbl)
              n118 = call <instrlib>:"Configure Multi Gate Parameters.vi"("error in (no error)"=w325, "Multi Gate Inspection"=w296, "Test Number"=w324) -> ("error out"=w321:errorcluster, "Test Number out"=w319:u32)  [unwired: 6 in, 1 out]
              n119 = Bundle By Name(cluster="Transmit Parameters 7", "Pulse Shape.Width"=w306, "Pulse Shape.Damping"=w305) -> (w295:T26)
              n120 = call <instrlib>:"Set Data Format.vi"("error in (no error)"=w321, "Data Formatting"="Data Formatting 7", "Test No."=w319) -> ("error out"=w323:errorcluster, "Test No. out"=w322:u32)  [unwired: 6 in, 1 out]
              n121 = call <instrlib>:"Configure Transmit Parameters.vi"("error in (no error)"=w323, "Transmit Parameters"=w295, "Tx Channel"=w322) -> ("error out"=w292:errorcluster)  [unwired: 7 in, 1 out]
            }
            frame "Channel 8" {
              n122 = call <instrlib>:"Add New Test.vi"("error in (no error)"=w339, "Test Parameters"=T30 {"Test No."=8, "Tx Channel"=8, "Rx Channel"=8}) -> ("error out"=w340:errorcluster, "Test No. out"=w336:u32)  [unwired: 6 in, 2 out]
              n123 = call <instrlib>:"Configure Receive Parameters.vi"("error in (no error)"=w340, "Receive Parameters"="Receive Parameters 8", "Test No."=w336) -> ("error out"=w345:errorcluster, "Test No. out"=w344:u32)  [unwired: 6 in, 1 out]
              n124 = call <instrlib>:"Configure Multi Gate Parameters.vi"("error in (no error)"=w345, "Multi Gate Inspection"="Multi Gate Inspection 8", "Test Number"=w344) -> ("error out"=w341:errorcluster, "Test Number out"=w335:u32)  [unwired: 6 in, 1 out]
              n125 = call <instrlib>:"Set Data Format.vi"("error in (no error)"=w341, "Data Formatting"="Data Formatting 8", "Test No."=w335) -> ("error out"=w343:errorcluster, "Test No. out"=w342:u32)  [unwired: 6 in, 1 out]
              n126 = call <instrlib>:"Configure Transmit Parameters.vi"("error in (no error)"=w343, "Transmit Parameters"="Transmit Parameters 8", "Tx Channel"=w342) -> ("error out"=w338:errorcluster)  [unwired: 7 in, 1 out]
            }
            frame "Channel 9" {
              n127 = call <instrlib>:"Add New Test.vi"("error in (no error)"=w360, "Test Parameters"=T30 {"Test No."=9, "Tx Channel"=9, "Rx Channel"=9}) -> ("error out"=w361:errorcluster, "Test No. out"=w358:u32)  [unwired: 6 in, 2 out]
              n128 = call <instrlib>:"Configure Receive Parameters.vi"("error in (no error)"=w361, "Receive Parameters"="Receive Parameters 9", "Test No."=w358) -> ("error out"=w366:errorcluster, "Test No. out"=w365:u32)  [unwired: 6 in, 1 out]
              n129 = call <instrlib>:"Configure Multi Gate Parameters.vi"("error in (no error)"=w366, "Multi Gate Inspection"="Multi Gate Inspection 9", "Test Number"=w365) -> ("error out"=w362:errorcluster, "Test Number out"=w357:u32)  [unwired: 6 in, 1 out]
              n130 = call <instrlib>:"Set Data Format.vi"("error in (no error)"=w362, "Data Formatting"="Data Formatting 9", "Test No."=w357) -> ("error out"=w364:errorcluster, "Test No. out"=w363:u32)  [unwired: 6 in, 1 out]
              n131 = call <instrlib>:"Configure Transmit Parameters.vi"("error in (no error)"=w364, "Transmit Parameters"="Transmit Parameters 9", "Tx Channel"=w363) -> ("error out"=w350:errorcluster)  [unwired: 7 in, 1 out]
              n132 = call <instrlib>:"Start Continuous Test Cycles [STP].vi"("error in (no error)"=w350) -> ("error out"=w349:errorcluster)  [unwired: 9 in, 1 out]
              n133 = call <instrlib>:"Force Gate Update On XY Chart.vi"("error in (no error)"=w349, "Test No."=u32 1) -> ("error out"=w348:errorcluster)  [unwired: 7 in, 2 out]
            }
          }
        }
      }
      frame "Main" {
        n134 = case shown="No Error" w374 {
          selector: w374 -> [w375 w620]
          tunnel: [w377 w620] -> w373
          tunnel: w372 -> [_ _]
          tunnel: [w376 TRUE ("NewVal")] -> w368
          frame No Error {
            n135 = while {
              tunnel: [w401] -> w376
              tunnel: [w401] -> _
              stop <- w401 stop-if-true
              n136 = event shown="[2] \"Channel 1 Interface\", \"Channel 2 Interface\", \"Channel 3 Interface\", \"Channel 4 Interface\", \"Channel 5 Interface\", \"Channel 6 Interface\", \"Channel 7 Interface\": Value Change" {
                selector: _ -> [_ _ _ _ _ _ _ _ _ _ _ _ _]
                dyn-events: _ -> [_ _ _ _ _ _ _ _ _ _ _ _ _]
                timeout: _ -> [_ _ _ _ _ _ _ _ _ _ _ _ _]
                tunnel: [FALSE ("NewVal") FALSE ("NewVal") _ _ _ _ _ _ _ _ FALSE ("NewVal") FALSE ("NewVal") w618] -> w401
                event Timeout {
                  n137 = event-data() -> ()  [unwired: 1 in, 3 out]
                }
                event "Channel Select": Value Change {
                  n138 = event-data() -> ("NewVal"=w407:u16)  [unwired: 1 in, 3 out]
                  n139 = property on="Channel Setup Tab Control" class="TabCtl (strict)"("Value"=w407) -> ()  [unwired: 2 in, 2 out]
                  n140 = case shown="6" w407 {
                    tunnel: [w412 w416 w420 w424 w428 w432 w436] -> w406
                    tunnel: [w410 w414 w418 w422 w426 w430 w434] -> w405
                    tunnel: [w409 w413 w417 w421 w425 w429 w433] -> w403
                    frame 0, Default {
                      n141 = property on="Channel 1 A-Scan Window" class="Clust (strict)"() -> ("Value"=w411:cluster{"Start":dbl, "Range":dbl})  [unwired: 2 in, 2 out]
                      n142 = Unbundle By Name(w411) -> ("Start"=w410:dbl, "Range"=w409:dbl)
                      n143 = property on="Gain" class="DigNum (strict)"() -> ("Value"=w412:dbl)  [unwired: 2 in, 2 out]
                    }
                    frame 1 {
                      n144 = property on="Channel 2 A-Scan Window" class="Clust (strict)"() -> ("Value"=w415:cluster{"Start":dbl, "Range":dbl})  [unwired: 2 in, 2 out]
                      n145 = Unbundle By Name(w415) -> ("Start"=w414:dbl, "Range"=w413:dbl)
                      n146 = property on="Gain" class="DigNum (strict)"() -> ("Value"=w416:dbl)  [unwired: 2 in, 2 out]
                    }
                    frame 2 {
                      n147 = property on="Channel 3 A-Scan Window" class="Clust (strict)"() -> ("Value"=w419:cluster{"Start":dbl, "Range":dbl})  [unwired: 2 in, 2 out]
                      n148 = Unbundle By Name(w419) -> ("Start"=w418:dbl, "Range"=w417:dbl)
                      n149 = property on="Gain" class="DigNum (strict)"() -> ("Value"=w420:dbl)  [unwired: 2 in, 2 out]
                    }
                    frame 3 {
                      n150 = property on="Channel 4 A-Scan Window" class="Clust (strict)"() -> ("Value"=w423:cluster{"Start":dbl, "Range":dbl})  [unwired: 2 in, 2 out]
                      n151 = Unbundle By Name(w423) -> ("Start"=w422:dbl, "Range"=w421:dbl)
                      n152 = property on="Gain" class="DigNum (strict)"() -> ("Value"=w424:dbl)  [unwired: 2 in, 2 out]
                    }
                    frame 4 {
                      n153 = property on="Channel 5 A-Scan Window" class="Clust (strict)"() -> ("Value"=w427:cluster{"Start":dbl, "Range":dbl})  [unwired: 2 in, 2 out]
                      n154 = Unbundle By Name(w427) -> ("Start"=w426:dbl, "Range"=w425:dbl)
                      n155 = property on="Gain" class="DigNum (strict)"() -> ("Value"=w428:dbl)  [unwired: 2 in, 2 out]
                    }
                    frame 5 {
                      n156 = property on="Channel 6 A-Scan Window" class="Clust (strict)"() -> ("Value"=w431:cluster{"Start":dbl, "Range":dbl})  [unwired: 2 in, 2 out]
                      n157 = Unbundle By Name(w431) -> ("Start"=w430:dbl, "Range"=w429:dbl)
                      n158 = property on="Gain" class="DigNum (strict)"() -> ("Value"=w432:dbl)  [unwired: 2 in, 2 out]
                    }
                    frame 6 {
                      n159 = property on="Channel 7 A-Scan Window" class="Clust (strict)"() -> ("Value"=w435:cluster{"Start":dbl, "Range":dbl})  [unwired: 2 in, 2 out]
                      n160 = Unbundle By Name(w435) -> ("Start"=w434:dbl, "Range"=w433:dbl)
                      n161 = property on="Gain" class="DigNum (strict)"() -> ("Value"=w436:dbl)  [unwired: 2 in, 2 out]
                    }
                  }
                  n162 = property on="Gain Slider" class="Slide (strict)"("Value"=w406) -> ()  [unwired: 2 in, 2 out]
                  n163 = Add(x=w405, y=w403) -> (x+y=w404:dbl)
                  n164 = property on="Channel Setup Graph" class="XYGraph (strict)"("XScale.Minimum"=w405, "XScale.Maximum"=w404) -> ()  [unwired: 2 in, 2 out]
                }
                event "Channel 1 Interface", "Channel 2 Interface", "Channel 3 Interface", "Channel 4 Interface", "Channel 5 Interface", "Channel 6 Interface", "Channel 7 Interface": Value Change {
                  (unwired) 2.0 ("y")
                  w446 = 1 ("Gate Number")
                  n165 = event-data() -> ("NewVal"=w444:T6)  [unwired: 1 in, 5 out]
                  n166 = Unbundle By Name(w444) -> ("Start"=w441:dbl, "Length"=w440:dbl, "Threshold"=w442:dbl)
                  n167 = property on="Velocity of Sound" class="DigNum (strict)"() -> ("Value"=w439:dbl)  [unwired: 2 in, 2 out]
                  n168 = call "DistanceToTime_mm_us.vi"("Length"=w440, "Start"=w441, "Value"=w439) -> ("Numeric"=w437:dbl, "Numeric 2"=w438:dbl)  [unwired: 7 in]
                  n169 = property on="Channel Select" class="Ring (strict)"() -> ("Value"=w443:u16)  [unwired: 2 in, 2 out]
                  n170 = Increment(x=w443) -> (x+1=w445:u16)
                  n171 = case shown="6" w443 {
                    tunnel: w437 -> [w449 w451 w455 w458 w461 w464 w467]
                    tunnel: w438 -> [w448 w452 w454 w457 w460 w463 w466]
                    tunnel: w442 -> [w447 w450 w453 w456 w459 w462 w465]
                    frame 0, Default {
                      n172 = property on="Length (us)" class="DigNum (strict)"("Value"=w448) -> ()  [unwired: 2 in, 2 out]
                      n173 = property on="Start (us)" class="DigNum (strict)"("Value"=w449) -> ()  [unwired: 2 in, 2 out]
                      n174 = property on="Threshold" class="DigNum (strict)"("Value"=w447) -> ()  [unwired: 2 in, 2 out]
                    }
                    frame 1 {
                      n175 = property on="Length (us)" class="DigNum (strict)"("Value"=w452) -> ()  [unwired: 2 in, 2 out]
                      n176 = property on="Start (us)" class="DigNum (strict)"("Value"=w451) -> ()  [unwired: 2 in, 2 out]
                      n177 = property on="Threshold" class="DigNum (strict)"("Value"=w450) -> ()  [unwired: 2 in, 2 out]
                    }
                    frame 2 {
                      n178 = property on="Length (us)" class="DigNum (strict)"("Value"=w454) -> ()  [unwired: 2 in, 2 out]
                      n179 = property on="Start (us)" class="DigNum (strict)"("Value"=w455) -> ()  [unwired: 2 in, 2 out]
                      n180 = property on="Threshold" class="DigNum (strict)"("Value"=w453) -> ()  [unwired: 2 in, 2 out]
                    }
                    frame 3 {
                      n181 = property on="Length (us)" class="DigNum (strict)"("Value"=w457) -> ()  [unwired: 2 in, 2 out]
                      n182 = property on="Start (us)" class="DigNum (strict)"("Value"=w458) -> ()  [unwired: 2 in, 2 out]
                      n183 = property on="Threshold" class="DigNum (strict)"("Value"=w456) -> ()  [unwired: 2 in, 2 out]
                    }
                    frame 4 {
                      n184 = property on="Length (us)" class="DigNum (strict)"("Value"=w460) -> ()  [unwired: 2 in, 2 out]
                      n185 = property on="Start (us)" class="DigNum (strict)"("Value"=w461) -> ()  [unwired: 2 in, 2 out]
                      n186 = property on="Threshold" class="DigNum (strict)"("Value"=w459) -> ()  [unwired: 2 in, 2 out]
                    }
                    frame 5 {
                      n187 = property on="Length (us)" class="DigNum (strict)"("Value"=w463) -> ()  [unwired: 2 in, 2 out]
                      n188 = property on="Start (us)" class="DigNum (strict)"("Value"=w464) -> ()  [unwired: 2 in, 2 out]
                      n189 = property on="Threshold" class="DigNum (strict)"("Value"=w462) -> ()  [unwired: 2 in, 2 out]
                    }
                    frame 6 {
                      n190 = property on="Length (us)" class="DigNum (strict)"("Value"=w466) -> ()  [unwired: 2 in, 2 out]
                      n191 = property on="Start (us)" class="DigNum (strict)"("Value"=w467) -> ()  [unwired: 2 in, 2 out]
                      n192 = property on="Threshold" class="DigNum (strict)"("Value"=w465) -> ()  [unwired: 2 in, 2 out]
                    }
                  }
                  n193 = call <instrlib>:"Set Multi Gate Timing[GMT].vi"("Gate Number"=w446, "Gate Length (us)"=w438, "Gate Start (us)"=w437, "Test Number"=w445) -> ()  [unwired: 6 in, 2 out]
                  n194 = call <instrlib>:"Set Multi Gate Threshold Level [UML].vi"("Gate Number"=w446, "Threshold"=w442, "Test Number"=w445) -> ()  [unwired: 7 in, 2 out]
                }
                event "Channel 1 Flaw Gate", "Channel 2 Flaw Gate", "Channel 3 Flaw Gate", "Channel 4 Flaw Gate", "Channel 5 Flaw Gate", "Channel 6 Flaw Gate", "Channel 7 Flaw Gate": Value Change {
                  w479 = 3 ("Gate Number")
                  n195 = event-data() -> ("NewVal"=w477:T6)  [unwired: 1 in, 5 out]
                  n196 = Unbundle By Name(w477) -> ("Start"=w468:dbl, "Length"=w470:dbl, "Threshold"=w471:dbl)
                  n197 = property on="Velocity of Sound" class="DigNum (strict)"() -> ("Value"=w474:dbl)  [unwired: 2 in, 2 out]
                  n198 = property on="Channel Select" class="Ring (strict)"() -> ("Value"=w476:u16)  [unwired: 2 in, 2 out]
                  n199 = Divide(x=w474, y=2.0) -> (x/y=w469:dbl)
                  n200 = Divide(x=w468, y=w469) -> (x/y=w473:dbl)
                  n201 = Divide(x=w470, y=w469) -> (x/y=w472:dbl)
                  n202 = Increment(x=w476) -> (x+1=w478:u16)
                  n203 = call <instrlib>:"Set Multi Gate Threshold Level [UML].vi"("Gate Number"=w479, "Threshold"=w471, "Test Number"=w478) -> ()  [unwired: 7 in, 2 out]
                  n204 = call <instrlib>:"Set Multi Gate Timing[GMT].vi"("Gate Number"=w479, "Gate Length (us)"=w472, "Gate Start (us)"=w473, "Test Number"=w478) -> ()  [unwired: 6 in, 2 out]
                  n205 = case shown="6" w476 {
                    tunnel: w473 -> [w482 w485 w488 w491 w494 w497 w500]
                    tunnel: w472 -> [w481 w484 w487 w490 w493 w496 w499]
                    tunnel: w471 -> [w480 w483 w486 w489 w492 w495 w498]
                    frame 0, Default {
                      n206 = property on="Start (us)" class="DigNum (strict)"("Value"=w482) -> ()  [unwired: 2 in, 2 out]
                      n207 = property on="Threshold" class="DigNum (strict)"("Value"=w480) -> ()  [unwired: 2 in, 2 out]
                      n208 = property on="Length (us)" class="DigNum (strict)"("Value"=w481) -> ()  [unwired: 2 in, 2 out]
                    }
                    frame 1 {
                      n209 = property on="Start (us)" class="DigNum (strict)"("Value"=w485) -> ()  [unwired: 2 in, 2 out]
                      n210 = property on="Threshold" class="DigNum (strict)"("Value"=w483) -> ()  [unwired: 2 in, 2 out]
                      n211 = property on="Length (us)" class="DigNum (strict)"("Value"=w484) -> ()  [unwired: 2 in, 2 out]
                    }
                    frame 2 {
                      n212 = property on="Start (us)" class="DigNum (strict)"("Value"=w488) -> ()  [unwired: 2 in, 2 out]
                      n213 = property on="Threshold" class="DigNum (strict)"("Value"=w486) -> ()  [unwired: 2 in, 2 out]
                      n214 = property on="Length (us)" class="DigNum (strict)"("Value"=w487) -> ()  [unwired: 2 in, 2 out]
                    }
                    frame 3 {
                      n215 = property on="Start (us)" class="DigNum (strict)"("Value"=w491) -> ()  [unwired: 2 in, 2 out]
                      n216 = property on="Threshold" class="DigNum (strict)"("Value"=w489) -> ()  [unwired: 2 in, 2 out]
                      n217 = property on="Length (us)" class="DigNum (strict)"("Value"=w490) -> ()  [unwired: 2 in, 2 out]
                    }
                    frame 4 {
                      n218 = property on="Start (us)" class="DigNum (strict)"("Value"=w494) -> ()  [unwired: 2 in, 2 out]
                      n219 = property on="Threshold" class="DigNum (strict)"("Value"=w492) -> ()  [unwired: 2 in, 2 out]
                      n220 = property on="Length (us)" class="DigNum (strict)"("Value"=w493) -> ()  [unwired: 2 in, 2 out]
                    }
                    frame 5 {
                      n221 = property on="Start (us)" class="DigNum (strict)"("Value"=w497) -> ()  [unwired: 2 in, 2 out]
                      n222 = property on="Threshold" class="DigNum (strict)"("Value"=w495) -> ()  [unwired: 2 in, 2 out]
                      n223 = property on="Length (us)" class="DigNum (strict)"("Value"=w496) -> ()  [unwired: 2 in, 2 out]
                    }
                    frame 6 {
                      n224 = property on="Start (us)" class="DigNum (strict)"("Value"=w500) -> ()  [unwired: 2 in, 2 out]
                      n225 = property on="Threshold" class="DigNum (strict)"("Value"=w498) -> ()  [unwired: 2 in, 2 out]
                      n226 = property on="Length (us)" class="DigNum (strict)"("Value"=w499) -> ()  [unwired: 2 in, 2 out]
                    }
                  }
                }
                event "Channel 1 Backwall Gate", "Channel 2 Backwall Gate", "Channel 3 Backwall Gate", "Channel 4 Backwall Gate", "Channel 5 Backwall Gate", "Channel 6 Backwall Gate", "Channel 7 Backwall Gate": Value Change {
                  w512 = 2 ("Gate Number")
                  n227 = event-data() -> ("NewVal"=w510:T6)  [unwired: 1 in, 5 out]
                  n228 = Unbundle By Name(w510) -> ("Start"=w502:dbl, "Length"=w503:dbl, "Threshold"=w508:dbl)
                  n229 = property on="Velocity of Sound" class="DigNum (strict)"() -> ("Value"=w507:dbl)  [unwired: 2 in, 2 out]
                  n230 = property on="Channel Select" class="Ring (strict)"() -> ("Value"=w509:u16)  [unwired: 2 in, 2 out]
                  n231 = Divide(x=w507, y=2.0) -> (x/y=w501:dbl)
                  n232 = Divide(x=w502, y=w501) -> (x/y=w505:dbl)
                  n233 = Divide(x=w503, y=w501) -> (x/y=w504:dbl)
                  n234 = Increment(x=w509) -> (x+1=w511:u16)
                  n235 = call <instrlib>:"Set Multi Gate Threshold Level [UML].vi"("Gate Number"=w512, "Threshold"=w508, "Test Number"=w511) -> ()  [unwired: 7 in, 2 out]
                  n236 = call <instrlib>:"Set Multi Gate Timing[GMT].vi"("Gate Number"=w512, "Gate Length (us)"=w504, "Gate Start (us)"=w505, "Test Number"=w511) -> ()  [unwired: 6 in, 2 out]
                  n237 = case shown="0, Default" w509 {
                    tunnel: w505 -> [w515 w518 w521 w524 w527 w530 w533]
                    tunnel: w504 -> [w514 w517 w520 w523 w526 w529 w532]
                    tunnel: w508 -> [w513 w516 w519 w522 w525 w528 w531]
                    frame 0, Default {
                      n238 = property on="Start (us)" class="DigNum (strict)"("Value"=w515) -> ()  [unwired: 2 in, 2 out]
                      n239 = property on="Length (us)" class="DigNum (strict)"("Value"=w514) -> ()  [unwired: 2 in, 2 out]
                      n240 = property on="Threshold" class="DigNum (strict)"("Value"=w513) -> ()  [unwired: 2 in, 2 out]
                    }
                    frame 1 {
                      n241 = property on="Start (us)" class="DigNum (strict)"("Value"=w518) -> ()  [unwired: 2 in, 2 out]
                      n242 = property on="Length (us)" class="DigNum (strict)"("Value"=w517) -> ()  [unwired: 2 in, 2 out]
                      n243 = property on="Threshold" class="DigNum (strict)"("Value"=w516) -> ()  [unwired: 2 in, 2 out]
                    }
                    frame 2 {
                      n244 = property on="Start (us)" class="DigNum (strict)"("Value"=w521) -> ()  [unwired: 2 in, 2 out]
                      n245 = property on="Length (us)" class="DigNum (strict)"("Value"=w520) -> ()  [unwired: 2 in, 2 out]
                      n246 = property on="Threshold" class="DigNum (strict)"("Value"=w519) -> ()  [unwired: 2 in, 2 out]
                    }
                    frame 3 {
                      n247 = property on="Start (us)" class="DigNum (strict)"("Value"=w524) -> ()  [unwired: 2 in, 2 out]
                      n248 = property on="Length (us)" class="DigNum (strict)"("Value"=w523) -> ()  [unwired: 2 in, 2 out]
                      n249 = property on="Threshold" class="DigNum (strict)"("Value"=w522) -> ()  [unwired: 2 in, 2 out]
                    }
                    frame 4 {
                      n250 = property on="Start (us)" class="DigNum (strict)"("Value"=w527) -> ()  [unwired: 2 in, 2 out]
                      n251 = property on="Length (us)" class="DigNum (strict)"("Value"=w526) -> ()  [unwired: 2 in, 2 out]
                      n252 = property on="Threshold" class="DigNum (strict)"("Value"=w525) -> ()  [unwired: 2 in, 2 out]
                    }
                    frame 5 {
                      n253 = property on="Start (us)" class="DigNum (strict)"("Value"=w530) -> ()  [unwired: 2 in, 2 out]
                      n254 = property on="Length (us)" class="DigNum (strict)"("Value"=w529) -> ()  [unwired: 2 in, 2 out]
                      n255 = property on="Threshold" class="DigNum (strict)"("Value"=w528) -> ()  [unwired: 2 in, 2 out]
                    }
                    frame 6 {
                      n256 = property on="Start (us)" class="DigNum (strict)"("Value"=w533) -> ()  [unwired: 2 in, 2 out]
                      n257 = property on="Length (us)" class="DigNum (strict)"("Value"=w532) -> ()  [unwired: 2 in, 2 out]
                      n258 = property on="Threshold" class="DigNum (strict)"("Value"=w531) -> ()  [unwired: 2 in, 2 out]
                    }
                  }
                }
                event "Channel 1 Filter/Rectification/VoS", "Channel 2 Filter/Rectification/VoS", "Channel 3 Filter/Rectification/VoS", "Channel 4 Filter/Rectification/VoS", "Channel 5 Filter/Rectification/VoS", "Channel 6 Filter/Rectification/VoS", "Channel 7 Filter/Rectification/VoS": Value Change {
                  n259 = event-data() -> ("NewVal"=w541:T5)  [unwired: 1 in, 5 out]
                  n260 = Unbundle By Name(w541) -> ("Filter"=w540:T4, "Enum"=w539:T31)
                  n261 = property on="Channel Select" class="Ring (strict)"() -> ("Value"=w535:u16)  [unwired: 2 in, 2 out]
                  n262 = case shown="0, Default" w535 {
                    selector: w535 -> [w542 w546 w550 w554 w558 w562 w566]
                    tunnel: w540 -> [w545 w549 w552 w555 w559 w564 w567]
                    tunnel: w539 -> [w544 w548 w551 w556 w560 w565 w568]
                    tunnel: [w543 w547 w553 w557 w561 w563 w569] -> w538
                    tunnel: [w542 w546 w550 w554 w558 w562 w566] -> w536
                    frame 0, Default {
                      n263 = property on="Bandpass" class="Enum (strict)"("Value"=w545) -> ()  [unwired: 2 in, 2 out]
                      n264 = property on="Waveform Type" class="Enum (strict)"("Value"=w544) -> ()  [unwired: 2 in, 2 out]
                      n265 = property on="Smoothing" class="DigNum (strict)"() -> ("Value"=w543:u16)  [unwired: 2 in, 2 out]
                    }
                    frame 1 {
                      n266 = property on="Bandpass" class="Enum (strict)"("Value"=w549) -> ()  [unwired: 2 in, 2 out]
                      n267 = property on="Waveform Type" class="Enum (strict)"("Value"=w548) -> ()  [unwired: 2 in, 2 out]
                      n268 = property on="Smoothing" class="DigNum (strict)"() -> ("Value"=w547:u16)  [unwired: 2 in, 2 out]
                    }
                    frame 2 {
                      n269 = property on="Bandpass" class="Enum (strict)"("Value"=w552) -> ()  [unwired: 2 in, 2 out]
                      n270 = property on="Waveform Type" class="Enum (strict)"("Value"=w551) -> ()  [unwired: 2 in, 2 out]
                      n271 = property on="Smoothing" class="DigNum (strict)"() -> ("Value"=w553:u16)  [unwired: 2 in, 2 out]
                    }
                    frame 3 {
                      n272 = property on="Bandpass" class="Enum (strict)"("Value"=w555) -> ()  [unwired: 2 in, 2 out]
                      n273 = property on="Waveform Type" class="Enum (strict)"("Value"=w556) -> ()  [unwired: 2 in, 2 out]
                      n274 = property on="Smoothing" class="DigNum (strict)"() -> ("Value"=w557:u16)  [unwired: 2 in, 2 out]
                    }
                    frame 4 {
                      n275 = property on="Bandpass" class="Enum (strict)"("Value"=w559) -> ()  [unwired: 2 in, 2 out]
                      n276 = property on="Waveform Type" class="Enum (strict)"("Value"=w560) -> ()  [unwired: 2 in, 2 out]
                      n277 = property on="Smoothing" class="DigNum (strict)"() -> ("Value"=w561:u16)  [unwired: 2 in, 2 out]
                    }
                    frame 5 {
                      n278 = property on="Bandpass" class="Enum (strict)"("Value"=w564) -> ()  [unwired: 2 in, 2 out]
                      n279 = property on="Waveform Type" class="Enum (strict)"("Value"=w565) -> ()  [unwired: 2 in, 2 out]
                      n280 = property on="Smoothing" class="DigNum (strict)"() -> ("Value"=w563:u16)  [unwired: 2 in, 2 out]
                    }
                    frame 6 {
                      n281 = property on="Bandpass" class="Enum (strict)"("Value"=w567) -> ()  [unwired: 2 in, 2 out]
                      n282 = property on="Waveform Type" class="Enum (strict)"("Value"=w568) -> ()  [unwired: 2 in, 2 out]
                      n283 = property on="Smoothing" class="DigNum (strict)"() -> ("Value"=w569:u16)  [unwired: 2 in, 2 out]
                    }
                  }
                  n284 = Increment(x=w536) -> (x+1=w534:u16)
                  n285 = call <instrlib>:"Set Waveform Type [AWF].vi"("Waveform Type"=w539, "Test Number"=w534) -> ("error out"=w537:errorcluster)  [unwired: 8 in, 1 out]
                  n286 = call <instrlib>:"Set Frequency Filter [FRQ].vi"("error in (no error)"=w537, "Smoothing"=w538, "Filter"=w540, "Test Number"=w534) -> ()  [unwired: 6 in, 2 out]
                }
                event "Channel 1 A-Scan Window", "Channel 2 A-Scan Window", "Channel 3 A-Scan Window", "Channel 4 A-Scan Window", "Channel 5 A-Scan Window", "Channel 6 A-Scan Window", "Channel 7 A-Scan Window": Value Change {
                  n287 = event-data() -> ("NewVal"=w576:cluster{"Start":dbl, "Range":dbl})  [unwired: 1 in, 5 out]
                  n288 = Unbundle By Name(w576) -> ("Start"=w579:dbl, "Range"=w578:dbl)
                  n289 = Unbundle By Name(w576) -> ("Start"=w582:dbl, "Range"=w581:dbl)
                  n290 = property on="Velocity of Sound" class="DigNum (strict)"() -> ("Value"=w572:dbl)  [unwired: 2 in, 2 out]
                  n291 = Add(x=w582, y=w581) -> (x+y=w580:dbl)
                  n292 = property on="Channel Select" class="Ring (strict)"() -> ("Value"=w584:u16)  [unwired: 2 in, 2 out]
                  n293 = Divide(x=w572, y=1.0) -> (x/y=w573:dbl)
                  n294 = property on="Channel Setup Graph" class="XYGraph (strict)"("XScale.Minimum"=w582, "XScale.Maximum"=w580, "XScale.Increment"=5.0 ("X Scale.Range:Increment")) -> ()  [unwired: 2 in, 2 out]
                  n295 = Divide(x=w579, y=w573) -> (x/y=w575:dbl)
                  n296 = Divide(x=w578, y=w573) -> (x/y=w574:dbl)
                  n297 = Increment(x=w584) -> (x+1=w583:u16)
                  n298 = Bundle By Name(cluster=w576, "Start"=w575, "Range"=w574) -> (w577:cluster{"Start":dbl, "Range":dbl})
                  n299 = call <instrlib>:"Set Inspection Gate [GAT].vi"("Gate Length (us)"=w574, "Gate Start (us)"=w575, "Test Number"=w583) -> ()  [unwired: 7 in, 2 out]
                  n300 = case shown="0, Default" w584 {
                    tunnel: w577 -> [w585 w586 w587 w588 w589 w590 w591]
                    frame 0, Default {
                      n301 = property on="Display Gate" class="Clust (strict)"("Value"=w585) -> ()  [unwired: 2 in, 2 out]
                    }
                    frame 1 {
                      n302 = property on="Display Gate" class="Clust (strict)"("Value"=w586) -> ()  [unwired: 2 in, 2 out]
                    }
                    frame 2 {
                      n303 = property on="Display Gate" class="Clust (strict)"("Value"=w587) -> ()  [unwired: 2 in, 2 out]
                    }
                    frame 3 {
                      n304 = property on="Display Gate" class="Clust (strict)"("Value"=w588) -> ()  [unwired: 2 in, 2 out]
                    }
                    frame 4 {
                      n305 = property on="Display Gate" class="Clust (strict)"("Value"=w589) -> ()  [unwired: 2 in, 2 out]
                    }
                    frame 5 {
                      n306 = property on="Display Gate" class="Clust (strict)"("Value"=w590) -> ()  [unwired: 2 in, 2 out]
                    }
                    frame 6 {
                      n307 = property on="Display Gate" class="Clust (strict)"("Value"=w591) -> ()  [unwired: 2 in, 2 out]
                    }
                  }
                }
                event "Channel 1 Filter/Rectification/VoS.Velocity of Sound", "Channel 2 Filter/Rectification/VoS.Velocity of Sound", "Channel 3 Filter/Rectification/VoS.Velocity of Sound", "Channel 4 Filter/Rectification/VoS.Velocity of Sound", "Channel 5 Filter/Rectification/VoS.Velocity of Sound", "Channel 6 Filter/Rectification/VoS.Velocity of Sound", "Channel 7 Filter/Rectification/VoS.Velocity of Sound": Value Change {
                  n308 = event-data() -> ("NewVal"=w592:dbl)  [unwired: 1 in, 5 out]
                  n309 = property on="Velocity of Sound" class="DigNum (strict)"("Value"=w592) -> ()  [unwired: 2 in, 2 out]
                  n310 = property on="Channel Setup Graph" class="XYGraph (strict)"("XScale.Multiplier"=w592) -> ()  [unwired: 2 in, 2 out]
                  n311 = property on="Velocity of Sound" class="DigNum (strict)"("Value"=w592) -> ()  [unwired: 2 in, 2 out]
                  n312 = property on="Velocity of Sound" class="DigNum (strict)"("Value"=w592) -> ()  [unwired: 2 in, 2 out]
                  n313 = property on="Velocity of Sound" class="DigNum (strict)"("Value"=w592) -> ()  [unwired: 2 in, 2 out]
                  n314 = property on="Velocity of Sound" class="DigNum (strict)"("Value"=w592) -> ()  [unwired: 2 in, 2 out]
                  n315 = property on="Velocity of Sound" class="DigNum (strict)"("Value"=w592) -> ()  [unwired: 2 in, 2 out]
                  n316 = property on="Velocity of Sound" class="DigNum (strict)"("Value"=w592) -> ()  [unwired: 2 in, 2 out]
                }
                event "Channel 1 PW & DAMP", "Channel 2 PW & DAMP", "Channel 3 PW & DAMP", "Channel 4 PW & DAMP", "Channel 5 PW & DAMP", "Channel 6 PW & DAMP", "Channel 7 PW & DAMP": Value Change {
                  n317 = event-data() -> ("NewVal"=w595:cluster{"Damping":T7, "Pulse Width":dbl})  [unwired: 1 in, 5 out]
                  n318 = Unbundle By Name(w595) -> ("Damping"=w594:T7, "Pulse Width"=w593:dbl)
                  n319 = property on="Channel Select" class="Ring (strict)"() -> ("Value"=w597:u16)  [unwired: 2 in, 2 out]
                  n320 = case shown="6" w597 {
                    tunnel: w595 -> [w598 w599 w600 w601 w602 w603 w604]
                    frame 0, Default {
                      n321 = property on="Pulse Shape" class="Clust (strict)"("Value"=w598) -> ()  [unwired: 2 in, 2 out]
                    }
                    frame 1 {
                      n322 = property on="Pulse Shape" class="Clust (strict)"("Value"=w599) -> ()  [unwired: 2 in, 2 out]
                    }
                    frame 2 {
                      n323 = property on="Pulse Shape" class="Clust (strict)"("Value"=w600) -> ()  [unwired: 2 in, 2 out]
                    }
                    frame 3 {
                      n324 = property on="Pulse Shape" class="Clust (strict)"("Value"=w601) -> ()  [unwired: 2 in, 2 out]
                    }
                    frame 4 {
                      n325 = property on="Pulse Shape" class="Clust (strict)"("Value"=w602) -> ()  [unwired: 2 in, 2 out]
                    }
                    frame 5 {
                      n326 = property on="Pulse Shape" class="Clust (strict)"("Value"=w603) -> ()  [unwired: 2 in, 2 out]
                    }
                    frame 6 {
                      n327 = property on="Pulse Shape" class="Clust (strict)"("Value"=w604) -> ()  [unwired: 2 in, 2 out]
                    }
                  }
                  n328 = Increment(x=w597) -> (x+1=w596:u16)
                  n329 = call <instrlib>:"Set Pulse Width and Damping [PDW].vi"("Width (ns)"=w593, "Damping"=w594, "Channel Number"=w596) -> ()  [unwired: 7 in, 2 out]
                }
                event "Gain Slider": Value Change {
                  n330 = event-data() -> ("NewVal"=w606:dbl)  [unwired: 1 in, 5 out]
                  n331 = property on="Channel Select" class="Ring (strict)"() -> ("Value"=w605:u16)  [unwired: 2 in, 2 out]
                  n332 = case shown="6" w605 {
                    tunnel: w606 -> [w608 w609 w610 w611 w612 w613 w614]
                    frame 0, Default {
                      n333 = property on="Gain" class="DigNum (strict)"("Value"=w608) -> ()  [unwired: 2 in, 2 out]
                    }
                    frame 1 {
                      n334 = property on="Gain" class="DigNum (strict)"("Value"=w609) -> ()  [unwired: 2 in, 2 out]
                    }
                    frame 2 {
                      n335 = property on="Gain" class="DigNum (strict)"("Value"=w610) -> ()  [unwired: 2 in, 2 out]
                    }
                    frame 3 {
                      n336 = property on="Gain" class="DigNum (strict)"("Value"=w611) -> ()  [unwired: 2 in, 2 out]
                    }
                    frame 4 {
                      n337 = property on="Gain" class="DigNum (strict)"("Value"=w612) -> ()  [unwired: 2 in, 2 out]
                    }
                    frame 5 {
                      n338 = property on="Gain" class="DigNum (strict)"("Value"=w613) -> ()  [unwired: 2 in, 2 out]
                    }
                    frame 6 {
                      n339 = property on="Gain" class="DigNum (strict)"("Value"=w614) -> ()  [unwired: 2 in, 2 out]
                    }
                  }
                  n340 = Increment(x=w605) -> (x+1=w607:u16)
                  n341 = call <instrlib>:"Set Gain [GAN].vi"("Gain (dB)"=w606, "Test Number"=w607) -> ()  [unwired: 8 in, 2 out]
                }
                event "MicroPulse Config Switch": Value Change {
                  n342 = event-data() -> ("NewVal"=w616:u16)  [unwired: 1 in, 3 out]
                  n343 = property on="MicroPulse SysDiag Tab" class="TabCtl (strict)"("Value"=w616) -> ()  [unwired: 2 in, 2 out]
                }
                event "Main Tab Control": Value Change {
                  n344 = event-data() -> ()  [unwired: 1 in, 4 out]
                }
                event "stop": Value Change {
                  n345 = event-data() -> ("NewVal"=w618:bool)  [unwired: 1 in, 3 out]
                }
              }
              n346 = Wait (ms)(milliseconds to wait=u32 100) -> ()  [unwired: 1 out]
            }
            n347 = control-ref of="Channel Setup Graph"() -> (w378:refnum<vi>)
            n348 = while {
              tunnel: w378 -> [w386]
              tunnel: [w384] -> w377
              tunnel: w375 -> [w381]
              stop <- w384 stop-if-true
              n349 = property on="Channel Select" class="Ring (strict)"() -> ("Value"=w380:u16)  [unwired: 2 in, 2 out]
              n350 = call <instrlib>:"Read MP Message.vi"("error in (no error)"=w381) -> ("error out"=w390:errorcluster, "scan data info"=w379:T32)  [unwired: 6 in, 3 out]
              n351 = Add(x=w380, y=u16 1) -> (x+y=w382:u16)
              n352 = call <instrlib>:"AScan+Peaks to XY Chart.vi"("error in (no error)"=w390, "scan data info"=w379, "Test No."=w382) -> ("error out"=w385:errorcluster, "Echo Range (us)"=w388:dbl, "AScan+Peaks"=w387:cluster{"timebase":dbl[], "data":u16[]}[], "Update Indicators?"=w389:bool)  [unwired: 3 in, 2 out]
              n353 = case shown="True" w389 {
                tunnel: w388 -> [_ w395]
                tunnel: w387 -> [_ w399]
                tunnel: w386 -> [_ w396]
                tunnel: w382 -> [_ w397]
                tunnel: [w391 w393] -> w384
                tunnel: w385 -> [w391 w398]
                frame False {
                }
                frame True {
                  n354 = call <instrlib>:"Adjust Peak Offsets On XY Chart.vi"("error in (no error)"=w398, "Echo Range in"=w395, "AScan+Peaks in"=w399) -> ("error out"=w394:errorcluster, "AScan+Peaks out"=→"Channel Setup Graph":cluster{"timebase":dbl[], "data":u16[]}[])  [unwired: 7 in]
                  n355 = call <instrlib>:"Draw Gates On XY Chart.vi"("error in (no error)"=w394, "Echo Range"=w395, "XYGraph in"=w396, "Test No."=w397) -> ("error out"=w393:errorcluster)  [unwired: 7 in]
                }
              }
            }
          }
          frame Error {
          }
        }
        n356 = Select(t=T29."Shutdown", s=w368, f=T29."Main") -> (s? t:f=w369:T29)
      }
      frame "Error" {
      }
      frame "Shutdown" {
      }
    }
  }
